vi "System und Gaseinstellung V2.vi"() -> ()   [LabVIEW 2020, in "System Einstellungen V2.lvlib"]
uses:
  System Einstellungen V2.lvlib
  Visualisierungs Elemente/String - Eingabefeld.ctl
  Gasflasche.ctl
  Gasflaschenkomponente.ctl
  Traegergas.ctl
  Visualisierungs Elemente/Button.ctl
  Optionen Eingabe.ctl
  Visualisierungs Elemente/Checkbox(boolsch).ctl
  Analysatoren.ctl
  Optionen.ctl
  Sprachverwaltung/FGV Aktion Tabelle zerlegen.ctl
  Passwortverwaltung/FGV Passwort Aktion.ctl
  Aktion FGV Gasbottledefinition.ctl
  Aktion FGV SystemEinstellungenV2.ctl
  Analysator Definition/FGV Analysator Definition Aktionen.ctl
  Aktioen FGV System.ctl
  AnalysatorDefinition.ctl
  Allgemein/allgemeine Sub-VIs.lvlib
  Sprachverwaltung/Sprachverwaltung.lvlib
  <vilib>/nisyscfg/nisyscfg.lvlib
  Passwortverwaltung/Passwort.lvlib
  Analysator Definition/Analysator Definition.lvlib
panel:
  in  "Registerkartenelement":T1(tab)
  in  "Werkseinstellung erstellen":T2 caption="Werkseinstellung"
  in  "Optionen Speichern":T2 caption="Speichern"
  in  "Neustart":T2
  in  "atm":dbl
  in  "mbar":dbl
  out "Zeit Steuerunge":timestamp caption="Aktuelle Zeit Steuerung:"
  out "Zeit Anlage":timestamp caption="Aktuelle Zeit Anlage:"
  in  "Systemzeit ändern":T2
  in  "Wartungsintervall:":sgl caption="Wartungsintervall" format="%#_5g"
  in  "Optionen":T3
  in  "Seriennummer":string caption="Seriennummer (fürs Protokoll)"
  in  "Type number (for Protocol)":string caption="Typennummer (fürs Protokoll)"
  in  "Analysator":T5="FT-IR"
  in  "Gasteiler Export":bool caption="Schaltfläche"
  in  "Gasteiler Importieren":bool caption="Schaltfläche"
  in  "Neuer Analysator":bool caption="Schaltfläche"
  in  "Name für Protokoll":string caption="Name (fürs Protokoll)"
  in  "Analysator löschen":bool caption="Schaltfläche"
  in  "Analysatoren Liste":i32(listbox) caption="Analyzer Definition"
  in  "Gasteiler Tabelle":i32(listbox) caption="Gas Divider Definition"
  in  "Neuer Gasteiler":bool caption="Schaltfläche"
  in  "Gasteiler Seriennummer":string caption="Seriennummer (fürs Protokoll)"
  in  "Gasteiler löschen":bool caption="Schaltfläche"
  in  "Gasteiler Type":string caption="Typennummer (fürs Protokoll)"
  in  "Gasteiler Name":string caption="Name"
  in  "Gasteiler Letzte Wartung":timestamp caption="Letzte Wartung" format="%<%d.%m.%Y>T"
  in  "Gasflaschenliste löschen":bool caption="Schaltfläche"
  in  "Gasflasche löschen":bool caption="Schaltfläche"
  in  "Gasflasche einfügen":bool caption="Schaltfläche"
  in  "Gasflasche ändern":bool caption="Schaltfläche"
  in  "Trägergas":T6="N2"
  in  "Komponente 5":T7={"Gasauswahl"="", "Konzentration IST"=0.0, "Einheit"="ppm", "Genauigkeit"=0.0} {"Konzentration IST" format="%#.4f"; "Genauigkeit" format="%#.1f"}
  in  "Komponente 4":T7={"Gasauswahl"="", "Konzentration IST"=0.0, "Einheit"="ppm", "Genauigkeit"=0.0} {"Konzentration IST" format="%#.4f"; "Genauigkeit" format="%#.1f"}
  in  "Komponente 3":T7={"Gasauswahl"="", "Konzentration IST"=0.0, "Einheit"="ppm", "Genauigkeit"=0.0} {"Konzentration IST" format="%#.4f"; "Genauigkeit" format="%#.1f"}
  in  "Komponente 2":T7={"Gasauswahl"="", "Konzentration IST"=0.0, "Einheit"="ppm", "Genauigkeit"=0.0} {"Konzentration IST" format="%#.4f"; "Genauigkeit" format="%#.1f"}
  in  "Komponente 1":T7={"Gasauswahl"="", "Konzentration IST"=0.0, "Einheit"="ppm", "Genauigkeit"=0.0} {"Konzentration IST" format="%#.4f"; "Genauigkeit" format="%#.1f"}
  in  "Gasflasche":T8={"Gasname für die Auswahl"="CH4", "Chargennummer"="D15442589", "Ablaufdatum"=timestamp(0 s since 1904-01-01)} {"Ablaufdatum" format="%<%d.%m.%Y>T"}
  in  "GF import":bool caption="Schaltfläche 2"
  in  "GF export":bool caption="Schaltfläche"
  in  "Gasflaschen Liste":i32(listbox)
  in  "Update Gas Selects":bool caption="Schaltfläche"
  in  "Gas Eingabe":T9 caption="Gasbezeichnung:"
  in  "Gas einfügen":bool caption="Schaltfläche"
  in  "Gas löschen":bool caption="Schaltfläche"
  in  "Gasauswahl":i32(listbox) caption="Gasauswahl:"
  # "Systemeinstellungen"
  # "Optionen"
  # "System Werkzeuge"
  # "Zeiteinstellung"
  # "Umrechner"
  # "Analysatorkonfiguration"
  # "Gasteilerkonfiguration"
  # "Gasflaschenkonfiguration"
  # "Gas"
  # "Konzentration"
  # "Einheit"
  # "Genauigkeit [%]"
  # "Gasflaschenliste"
  # "Gasdefinition"
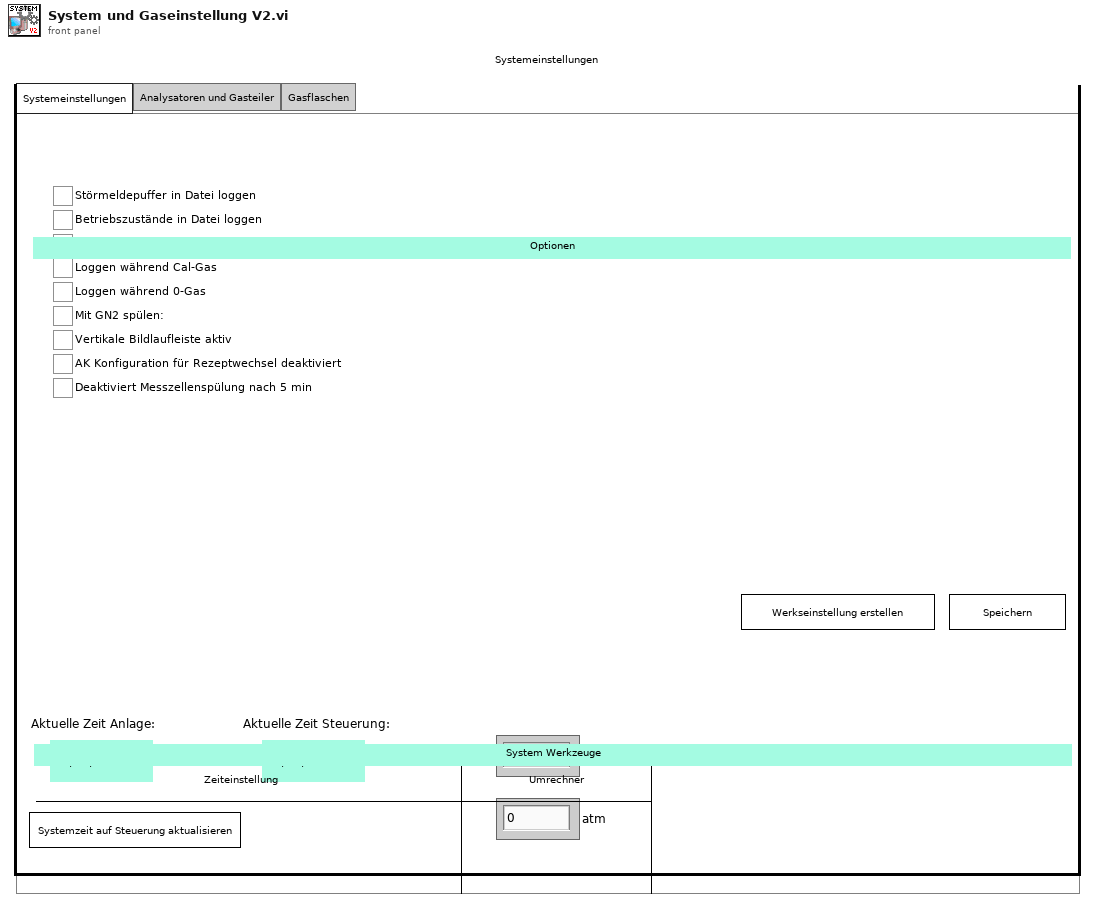
[diagram p1: front panel]
types:
  T1 = enum32{"Systemeinstellungen", "Analysatoren", "Gasflaschenkonfiguration", "Gasdefinition"}
  T2 = typedef "Button.ctl" = bool
  T3 = typedef "System Einstellungen V2.lvlib/Optionen Eingabe.ctl" = cluster{"Option 1":T4, "Option 2":T4, "Option 3":T4, "Option 4":T4, "Option 5":T4, "Option 6":T4, "Option 7":T4, "Option 8":T4, "Option 9":T4, "Option 10":T4, "Option 11":T4, "Option 12":T4, "Option 13":T4, "Option 14":T4, "Option 15":T4, "Option 16":T4, "Option 17":T4, "Option 18":T4, "Option 19":T4, "Option 20":T4, "Option 21":T4, "Option 22":T4, "Option 23":T4, "Option 24":T4, "Option 25":T4, "Option 26":T4, "Option 27":T4, "Option 28":T4, "Option 29":T4, "Option 30":T4, "Option 31":T4, "Option 32":T4, "Option 33":T4, "Option 34":T4, "Option 35":T4, "Option 36":T4, "Option 37":T4, "Option 38":T4, "Option 39":T4, "Option 40":T4, "Option 41":T4, "Option 42":T4, "Option 43":T4, "Option 44":T4, "Option 45":T4, "Option 46":T4, "Option 47":T4, "Option 48":T4, "Option 49":T4, "Option 50":T4, "Option 51":T4, "Option 52":T4, "Option 53":T4, "Option 54":T4, "Option 55":T4, "Option 56":T4, "Option 57":T4, "Option 58":T4, "Option 59":T4, "Option 60":T4}
  T4 = typedef "Checkbox(boolsch).ctl" = bool
  T5 = typedef "System Einstellungen V2.lvlib/Analysatoren.ctl" = string
  T6 = typedef "System Einstellungen V2.lvlib/Traegergas.ctl" = string
  T7 = typedef "System Einstellungen V2.lvlib/Gasflaschenkomponente.ctl" = cluster{"Gasauswahl":string, "Konzentration IST":dbl, "Einheit":string, "Genauigkeit":dbl}
  T8 = typedef "System Einstellungen V2.lvlib/Gasflasche.ctl" = cluster{"Gasname für die Auswahl":string, "Chargennummer":string, "Ablaufdatum":timestamp}
  T9 = typedef "String - Eingabefeld.ctl" = string
  T10 = typedef "Sprachverwaltung.lvlib/FGV Aktion Tabelle zerlegen.ctl" = enum16{"laden", "vereinzeln", "speichern"}
  T11 = enum8{"Enabled", "Disabled", "Disabled and Grayed Out"}
  T12 = typedef "Passwort.lvlib/FGV Passwort Aktion.ctl" = enum16{"prüfen", "setzen", "Initialisieren", "PW speichern", "lesen", "PW Änderung"}
  T13 = typedef "System Einstellungen V2.lvlib/Aktion FGV Gasbottledefinition.ctl" = enum16{"lesen", "schreiben", "löschen", "laden", "speichern", "exportieren", "importieren"}
  T14 = enum16{"lesen", "schreiben", "löschen", "laden", "speichern"}
  T15 = typedef "Analysator Definition.lvlib/FGV Analysator Definition Aktionen.ctl" = enum16{"lesen", "MB setzen", "MB KAL setzen", "laden"}
  T16 = typedef "System Einstellungen V2.lvlib/Aktion FGV SystemEinstellungenV2.ctl" = enum16{"lesen", "Analysatoren schreiben", "Analysator ändern", "Analysatoren löschen", "laden", "speichern", "Untertitel", "Analysatoren", "Neue Analysatoren", "Gasteiler schreiben", "Gasteiler ändern", "Gasteiler löschen", "Gasteiler", "Gasteiler exportieren", "Gasteiler importieren"}
  T17 = typedef "System Einstellungen V2.lvlib/Aktioen FGV System.ctl" = enum16{"lesen", "laden", "speichern", "Optionen schreiben", "Zeitstempel", "Reset BMP", "Reset SQP", "Wartung", "Werkseinstellung"}
  T18 = typedef "System Einstellungen V2.lvlib/Optionen.ctl" = cluster{"Störmeldep.":bool, "Betriebszustände":bool, "AK in ppm":bool, "log Cal-Gas":bool, "log 0-Gas":bool, "Durchflusssensor 0-5V":bool, "PNS?":bool, "Mit N2 spülen":bool, "TRE08":bool, "Amium 10-Fach":bool, "Verticale Scrollbar aktiv":bool, "Loggingtakt":bool, "AK Rezeptwechsel gleich wie MKS":bool, "NG ECO":bool}
  T19 = typedef "System Einstellungen V2.lvlib/Gasteiler.ctl" = cluster{"Gasteiler Name":string, "Gasteiler Type":string, "Gasteiler Seriennummer":string, "Gasteiler Letzte Wartung":timestamp}
  T20 = cluster{"GasteilerDefinitionsListe":T19[], "GasteilerDefinitionTextliste":string[][], "Gasteiler Strings And Values":cluster{"String":string, "Wert":string}[]}
  T21 = typedef "System Einstellungen V2.lvlib/AnalysatorDefinition.ctl" = cluster{"Analysator":string, "Name für Protokoll":string, "Type":string, "Seriennummer":string}
  T22 = typedef "LVComboBoxStrsAndValuesArrayTypeDef.ctl" = cluster{"String":string, "Value":string}[]
  T23 = cluster{"AnalysatorDefinitionListe":T21[], "AnalysatorDefinitionTextListe":string[][], "Analysatoren Strings And Values[]":T22}
  T24 = cluster{"Gasteiler Name":string, "Gasteiler Type":string, "Gasteiler Seriennummer":string, "Gasteiler Letzte Wartung":timestamp}
  T25 = typedef "System Einstellungen V2.lvlib/Gasflasche gesamt.ctl" = cluster{"Gasflasche":T8, "Trägergas":T6, "Komponenten":T7[]}
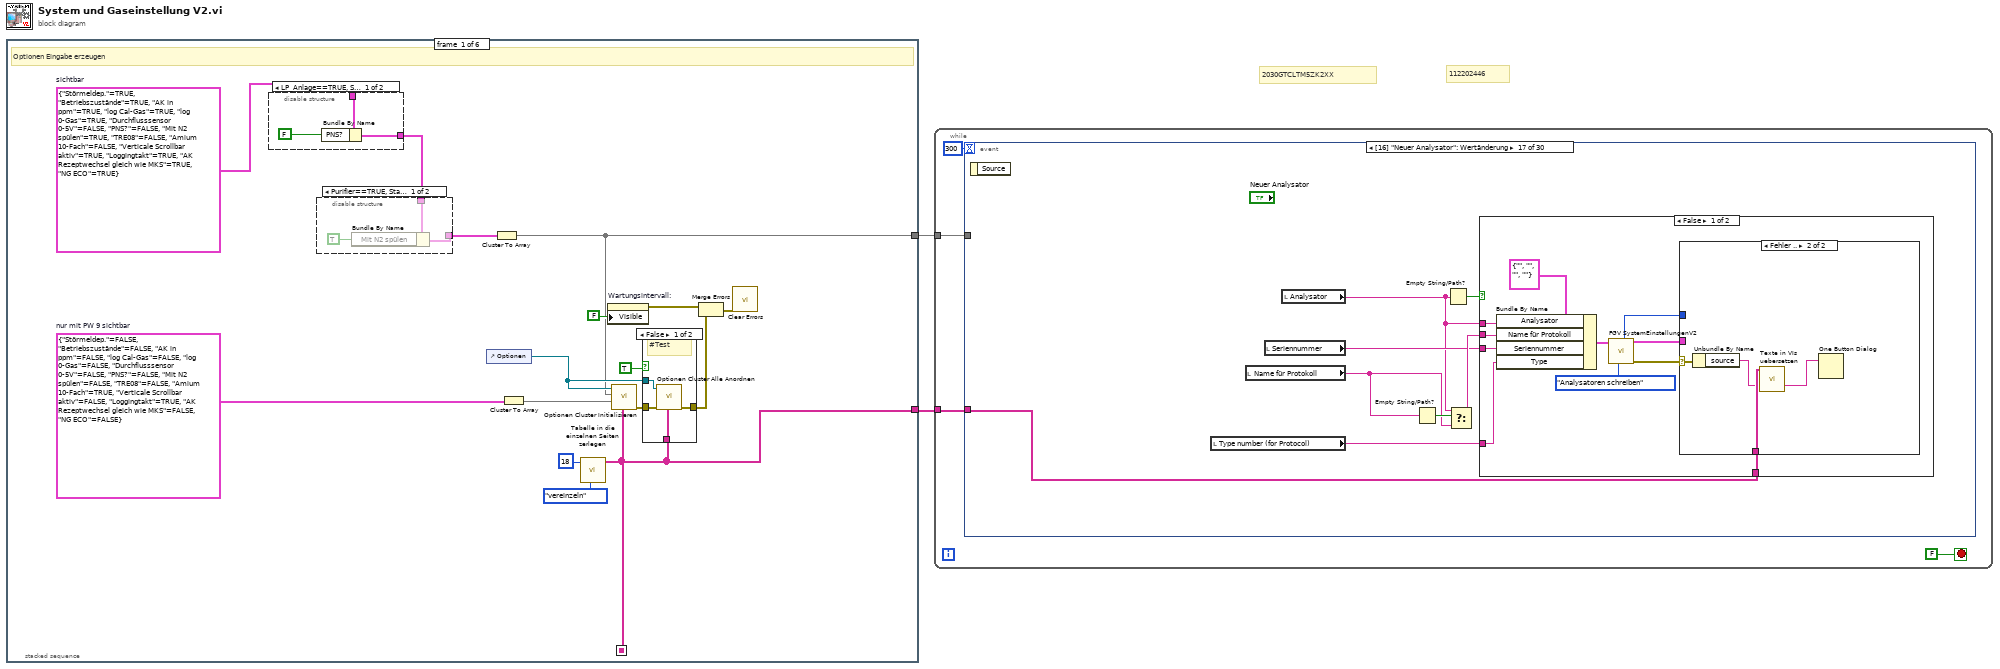
[diagram p0: block diagram]
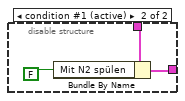
[diagram p2: hidden frame]
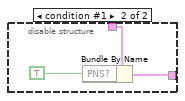
[diagram p3: hidden frame]
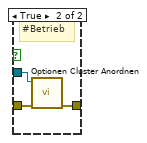
[diagram p4: hidden frame]
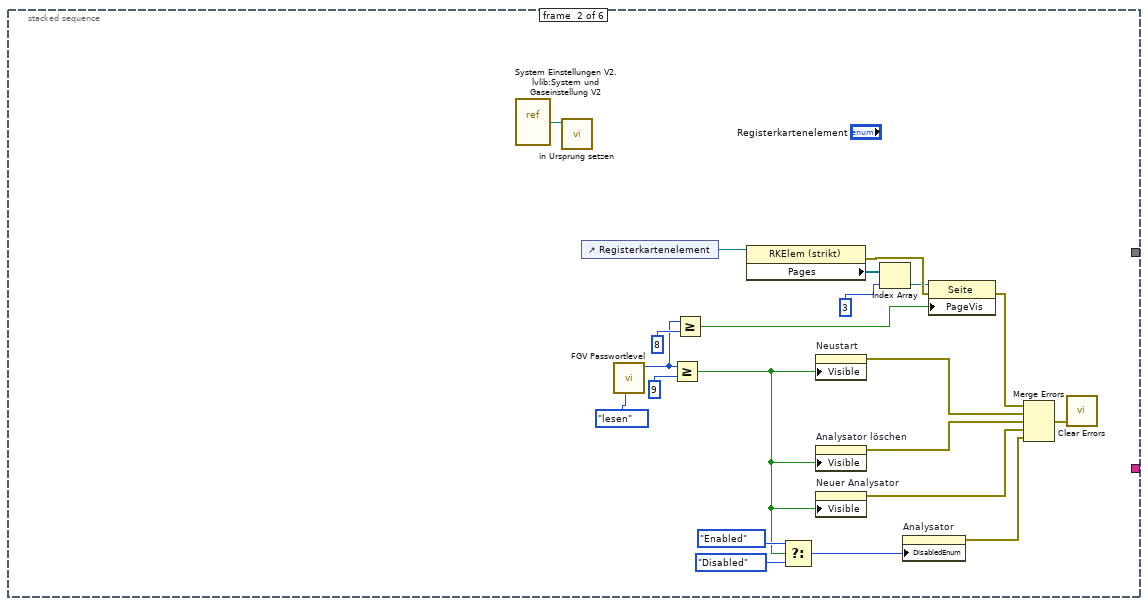
[diagram p5: hidden frame]
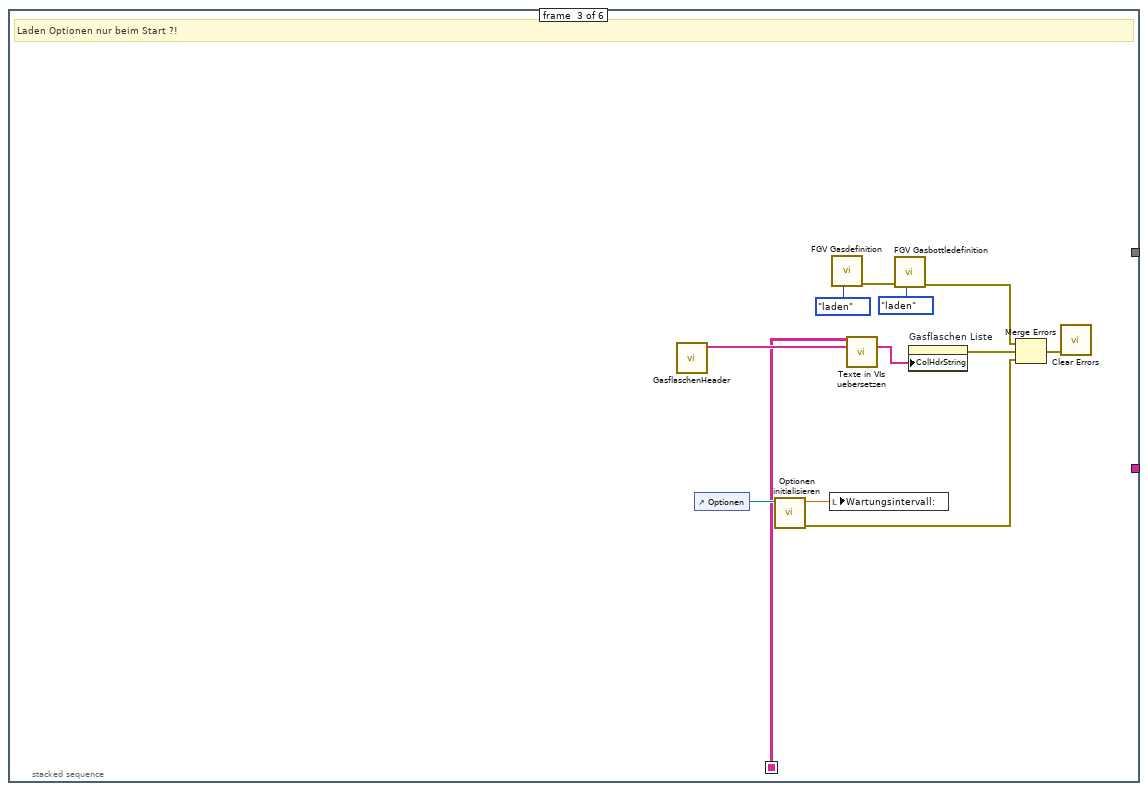
[diagram p6: hidden frame]
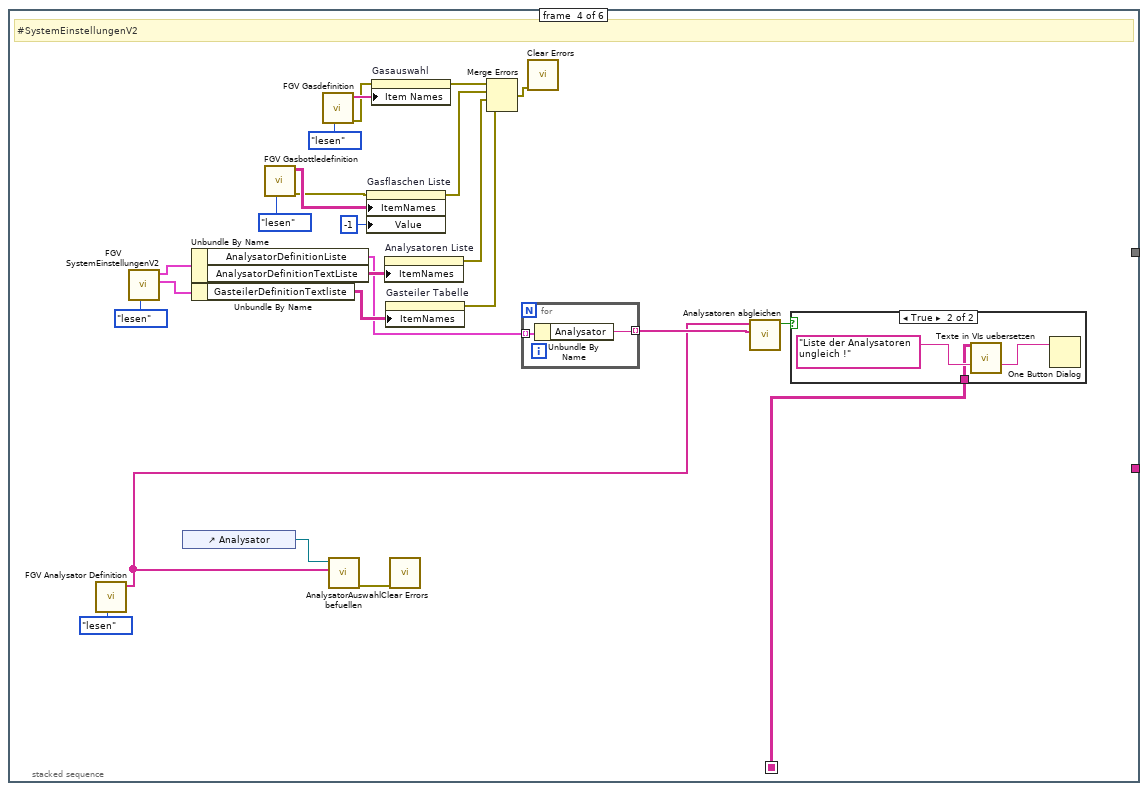
[diagram p7: hidden frame]
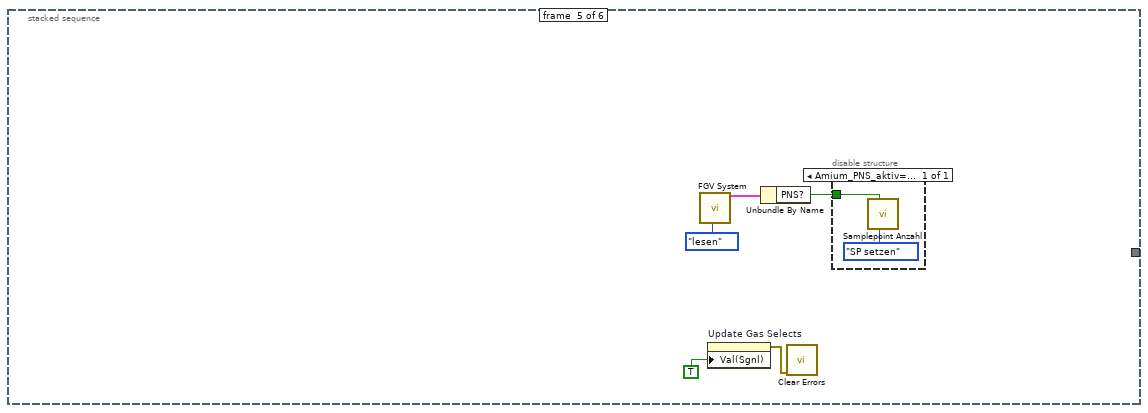
[diagram p9: hidden frame]
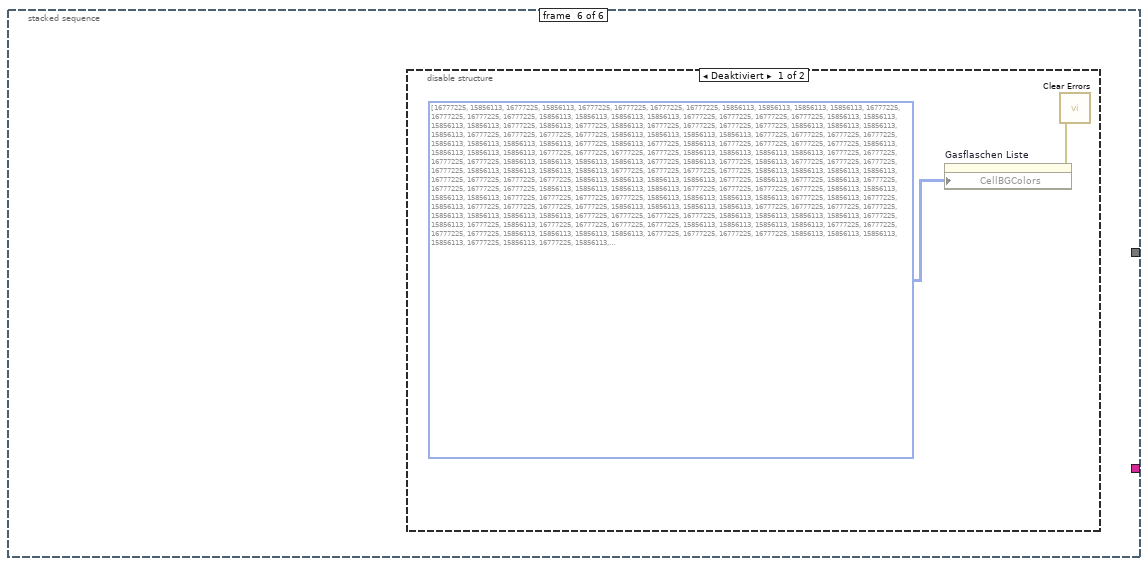
[diagram p10: hidden frame]
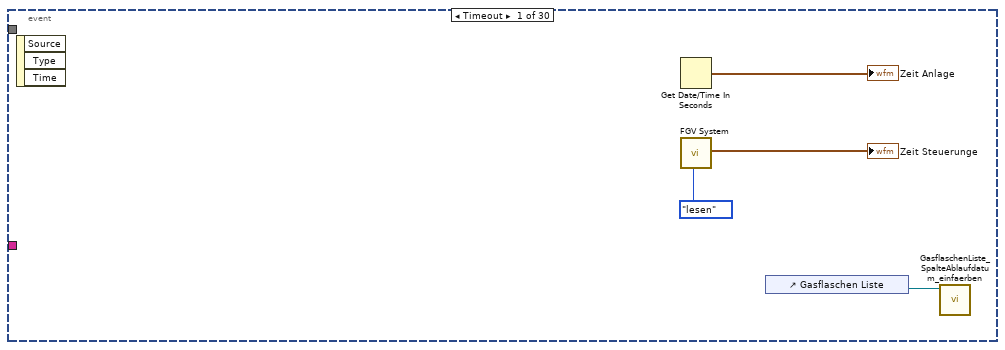
[diagram p12: hidden frame]
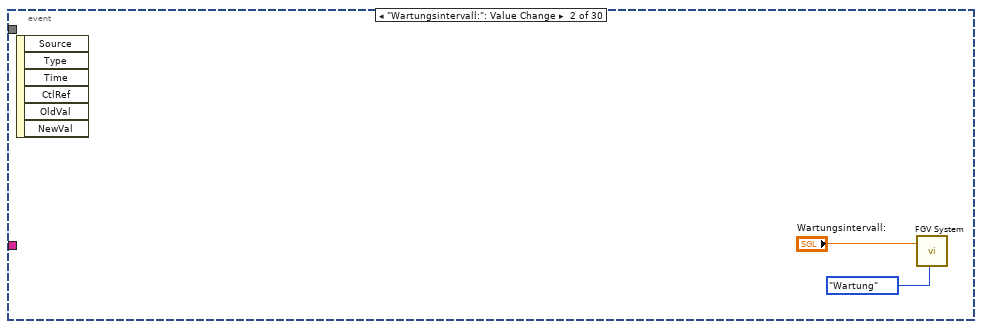
[diagram p13: hidden frame]
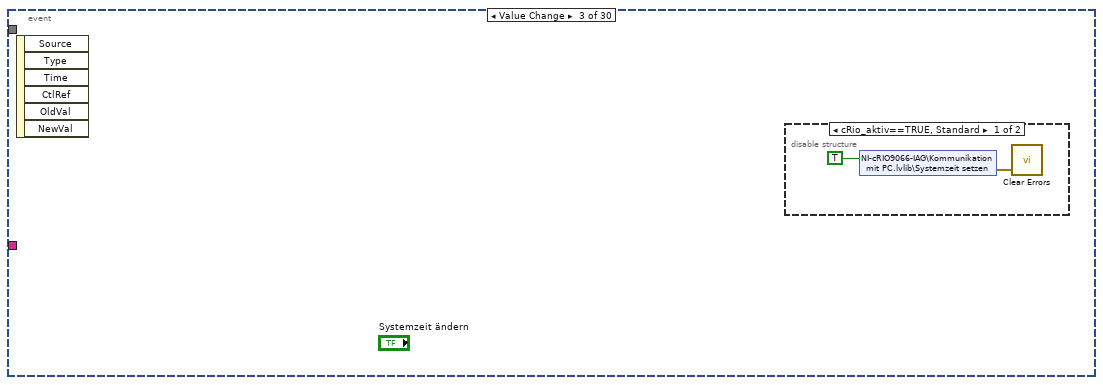
[diagram p14: hidden frame]
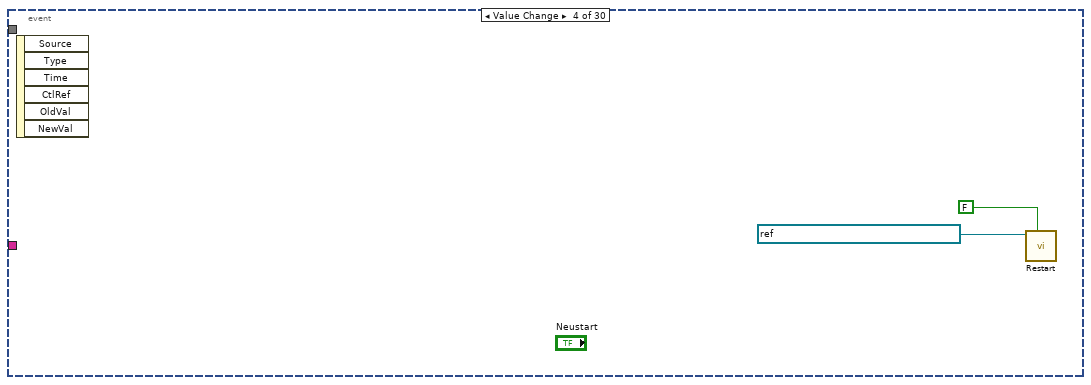
[diagram p16: hidden frame]
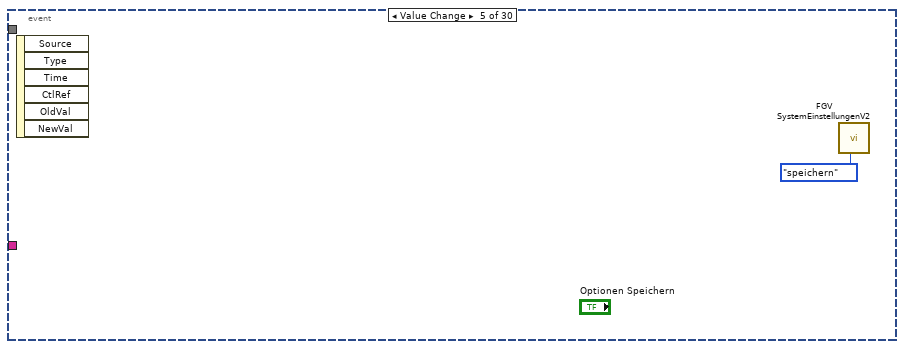
[diagram p17: hidden frame]
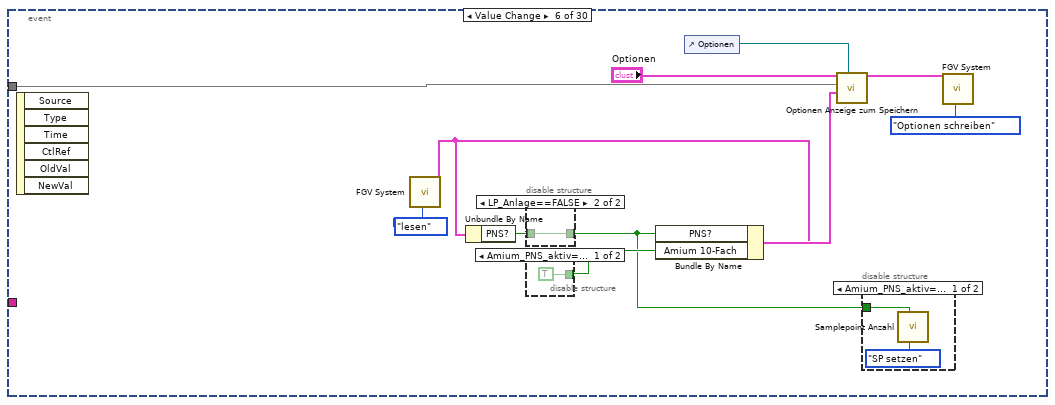
[diagram p18: hidden frame]
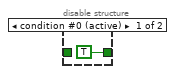
[diagram p19: hidden frame]
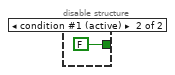
[diagram p20: hidden frame]
diagram:
  # "112202446"
  # "2030GTCLTM5ZK2XX"
  n1 = stacked-sequence {
    seq-local: [w3 _ _ _ _ _] -> [_ _ w59 w71 _ _]
    tunnel: [w14 _ _ _ _ _] -> w2
    tunnel: [w3 _ _ _ _ _] -> w1
    frame #0 {
      w12 = T18 {"Störmeldep."=FALSE, "Betriebszustände"=FALSE, "AK in ppm"=FALSE, "log Cal-Gas"=FALSE, "log 0-Gas"=FALSE, "Durchflusssensor 0-5V"=FALSE, "PNS?"=FALSE, "Mit N2 spülen"=FALSE, "TRE08"=FALSE, "Amium 10-Fach"=TRUE, "Verticale Scrollbar aktiv"=FALSE, "Loggingtakt"=TRUE, "AK Rezeptwechsel gleich wie MKS"=FALSE, "NG ECO"=FALSE}  # nur mit PW 9 sichtbar
      w11 = T18 {"Störmeldep."=TRUE, "Betriebszustände"=TRUE, "AK in ppm"=TRUE, "log Cal-Gas"=TRUE, "log 0-Gas"=TRUE, "Durchflusssensor 0-5V"=FALSE, "PNS?"=FALSE, "Mit N2 spülen"=TRUE, "TRE08"=FALSE, "Amium 10-Fach"=FALSE, "Verticale Scrollbar aktiv"=TRUE, "Loggingtakt"=TRUE, "AK Rezeptwechsel gleich wie MKS"=TRUE, "NG ECO"=TRUE}  # sichtbar
      # "Optionen Eingabe erzeugen"
      n2 = disable-structure shown="LP_Anlage==TRUE, Standard" {
        disable-tunnel: w11 -> [w27 w28]
        disable-tunnel: [w25 w29] -> w10
        frame condition #0 (active) {
          n3 = Bundle By Name(cluster=w27, "PNS?"=FALSE ("Störmeldepuffer")) -> (w25:T18)
        }
        frame condition #1 {
          n4 = Bundle By Name(cluster=w28, "PNS?"=TRUE ("Störmeldepuffer")) -> (w29:T18)
        }
      }
      n5 = disable-structure shown="Purifier==TRUE, Standard" {
        disable-tunnel: w10 -> [w21 w23]
        disable-tunnel: [w19 w22] -> w9
        frame condition #0 {
          n6 = Bundle By Name(cluster=w21, "Mit N2 spülen"=TRUE ("Störmeldepuffer")) -> (w19:T18)
        }
        frame condition #1 (active) {
          n7 = Bundle By Name(cluster=w23, "Mit N2 spülen"=FALSE ("Störmeldepuffer")) -> (w22:T18)
        }
      }
      n8 = control-ref of="Optionen"() -> (w17:refnum<vi>)
      n9 = Cluster To Array(cluster=w9) -> (array=w14:bool[])
      n10 = Cluster To Array(cluster=w12) -> (array=w13:bool[])
      n11 = call "Tabelle in die einzelnen Seiten zerlegen.vi"("Aktion"=FGV_Aktion_Tabelle_zerlegen."vereinzeln", "Index (Seite)"=18) -> ("Sprachliste"=w3:string[][])  [unwired: 7 in, 2 out]
      n12 = property on="Wartungsintervall:" class="DigWert (strikt)"("Visible"=FALSE ("Sichtbar")) -> (error out=w8:errorcluster)  [unwired: 2 in, 1 out]
      n13 = call "Optionen Cluster Initialisieren.vi"("Sprachliste"=w3, "PWL9"=w13, "sichtbar"=w14, "Cluster (Eingang)"=w17) -> ("error out"=w16:errorcluster)  [unwired: 5 in, 2 out]
      n14 = case shown="False" TRUE {
        tunnel: w17 -> [w32 w37]
        tunnel: w16 -> [w34 w36]
        tunnel: [w33 w35] -> w7
        tunnel: w3 -> [w31 _]
        frame False {
          # "#Test"
          n15 = call "Optionen Cluster Alle Anordnen.vi"("Sprachliste"=w31, "error in (no error)"=w34, "Cluster (Eingang)"=w32) -> ("error out"=w33:errorcluster)  [unwired: 7 in, 1 out]
        }
        frame True {
          # "#Betrieb"
          n16 = call "Optionen Cluster Anordnen.vi"("error in (no error)"=w36, "Cluster (Eingang)"=w37) -> ("error out"=w35:errorcluster)  [unwired: 8 in, 1 out]
        }
      }
      n17 = Merge Errors(w8, w7) -> (w6:errorcluster)
      n18 = call <vilib>:"Clear Errors.vi"("error in (no error)"=w6) -> ()  [unwired: 5 in, 2 out]
    }
    frame #1 {
      n19 = vi-ref "System Einstellungen V2.lvlib:System und Gaseinstellung V2.vi"() -> (w58:refnum<vi>)
      n20 = call "in Ursprung setzen.vi"("VI Referenz"=w58) -> ()  [unwired: 10 in, 1 out]
      n21 = control-ref of="Registerkartenelement"() -> (w52:refnum<vi>)
      n22 = call "FGV Passwortlevel.vi"("FGV Passwort Aktion"=FGV_Passwort_Aktion."lesen") -> ("aktueller Level"=w41:i16)  [unwired: 8 in, 2 out]
      n23 = Greater Or Equal?(x=w41, y=i16 9) -> (x >= y?=w43:bool)
      n24 = Greater Or Equal?(x=w41, y=i16 8) -> (x >= y?=w40:bool)
      n25 = property class="RKElem (strikt)"(reference=w52) -> (error out=w55:errorcluster, "Pages"=w54:refnum<vi>[])  [unwired: 1 in, 1 out]
      n26 = Select(t=T11."Enabled" ("Deaktiviert"), s=w43, f=T11."Disabled") -> (s? t:f=w39:T11)
      n27 = property on="Neustart" class="Bool."("Visible"=w43) -> (error out=w50:errorcluster)  [unwired: 2 in, 1 out]
      n28 = property on="Analysator löschen" class="Bool."("Visible"=w43) -> (error out=w47:errorcluster)  [unwired: 2 in, 1 out]
      n29 = property on="Neuer Analysator" class="Bool."("Visible"=w43) -> (error out=w46:errorcluster)  [unwired: 2 in, 1 out]
      n30 = Index Array(array=w54, index=3 ("Index")) -> (element=w53:refnum<vi>)
      n31 = property on="Analysator" class="KombiFeld (strikt)"("DisabledEnum"=w39) -> (error out=w38:errorcluster)  [unwired: 2 in, 1 out]
      n32 = property class="Seite"(reference=w53, error in=w55, "PageVis"=w40) -> (error out=w49:errorcluster)  [unwired: 1 out]
      n33 = Merge Errors(w49, w50, w47, w46, w38) -> (w48:errorcluster)
      n34 = call <vilib>:"Clear Errors.vi"("error in (no error)"=w48) -> ()  [unwired: 5 in, 2 out]
    }
    frame #2 {
      # "Laden Optionen nur beim Start ?!"
      n35 = call "GasflaschenHeader.vi"() -> ("Header"=w67:string[])  [unwired: 10 in, 1 out]
      n36 = control-ref of="Optionen"() -> (w65:refnum<vi>)
      n37 = call "Optionen initialisieren.vi"("Cluster (Eingang)"=w65) -> ("Fehler (Ausgang)"=w62:errorcluster, "Wartungsintervall:"=w64:sgl)  [unwired: 9 in]
      n38 = local write "Wartungsintervall:"(w64) -> ()
      n39 = call "FGV Gasdefinition.vi"("Aktion"=T14."laden") -> ("error out"=w68:errorcluster)  [unwired: 9 in, 1 out]
      n40 = call "Texte in VIs uebersetzen.vi"("Sprachliste"=w59, "String-Array zum Übersetzen"=w67) -> ("String-Array zum Übersetzen"=w66:string[])  [unwired: 9 in, 4 out]
      n41 = call "FGV Gasbottledefinition.vi"("Aktion"=Aktion_FGV_Gasbottledefinition."laden", "error in (no error)"=w68) -> ("error out"=w61:errorcluster)  [unwired: 7 in, 2 out]
      n42 = property on="Gasflaschen Liste" class="MehrSpaltFeld (strikt)"("ColHdrString"=w66) -> (error out=w63:errorcluster)  [unwired: 2 in, 1 out]
      n43 = Merge Errors(w61, w63, w62) -> (w60:errorcluster)
      n44 = call <vilib>:"Clear Errors.vi"("error in (no error)"=w60) -> ()  [unwired: 5 in, 2 out]
    }
    frame #3 {
      # "#SystemEinstellungenV2"
      n45 = call "FGV Analysator Definition.vi"("Aktionen"=FGV_Analysator_Definition_Aktionen."lesen") -> ("Analysatoren"=w72:string[])  [unwired: 6 in, 4 out]
      n46 = call "FGV SystemEinstellungenV2.vi"("Aktion"=Aktion_FGV_SystemEinstellungenV2."lesen") -> ("Gasteiler"=w85:T20, "Analysatoren"=w86:T23)  [unwired: 5 in, 4 out]
      n47 = control-ref of="Analysator"() -> (w75:refnum<vi>)
      n48 = Unbundle By Name(w86) -> ("AnalysatorDefinitionListe"=w83:T21[], "AnalysatorDefinitionTextListe"=w87:string[][])
      n49 = Unbundle By Name(w85) -> ("GasteilerDefinitionTextliste"=w84:string[][])
      n50 = call "FGV Gasbottledefinition.vi"("Aktion"=Aktion_FGV_Gasbottledefinition."lesen") -> ("error out"=w91:errorcluster, "Gasflaschen Text Liste gesamt"=w92:T6[][])  [unwired: 8 in, 1 out]
      n51 = call "FGV Gasdefinition.vi"("Aktion"=T14."lesen") -> ("error out"=w90:errorcluster, "Gase"=w94:string[])  [unwired: 9 in]
      n52 = call "AnalysatorAuswahl befuellen.vi"("Analysatoren"=w72, "Analysator Definition (Eingang)"=w75) -> ("error out"=w76:errorcluster)  [unwired: 9 in]
      n53 = property on="Gasflaschen Liste" class="MehrSpaltFeld (strikt)"(error in=w91, "ItemNames"=w92, "Value"=-1 ("Gasflaschen Liste")) -> (error out=w79:errorcluster)  [unwired: 1 in, 1 out]
      n54 = property on="Gasauswahl" class="Listenfeld (strikt)"(error in=w90, "Item Names"=w94) -> (error out=w81:errorcluster)  [unwired: 1 in, 1 out]
      n55 = property on="Analysatoren Liste" class="MehrSpaltFeld (strikt)"("ItemNames"=w87) -> (error out=w78:errorcluster)  [unwired: 2 in, 1 out]
      n56 = property on="Gasteiler Tabelle" class="MehrSpaltFeld (strikt)"("ItemNames"=w84) -> (error out=w77:errorcluster)  [unwired: 2 in, 1 out]
      n57 = call <vilib>:"Clear Errors.vi"("error in (no error)"=w76) -> ()  [unwired: 5 in, 2 out]
      n58 = Merge Errors(w81, w79, w78, w77) -> (w80:errorcluster)
      n59 = for {
        tunnel: w83 -> [w100] mode=indexing
        tunnel: [w99] -> w82 mode=indexing
        n60 = Unbundle By Name(w100) -> ("Analysator"=w99:string)
      }
      n61 = call <vilib>:"Clear Errors.vi"("error in (no error)"=w80) -> ()  [unwired: 5 in, 2 out]
      n62 = call "Analysatoren abgleichen.vi"("Analysatorliste"=w82, "Analysatoren"=w72) -> ("x != y?"=w73:bool)  [unwired: 9 in]
      n63 = case shown="True" w73 {
        tunnel: w71 -> [_ w96]
        frame False {
        }
        frame True {
          n64 = call "Texte in VIs uebersetzen.vi"("Sprachliste"=w96, "String zum Übersetzen"="Liste der Analysatoren ungleich !" ("Nachricht")) -> ("String zum Übersetzen"=w97:string)  [unwired: 9 in, 4 out]
          n65 = One Button Dialog(message=w97) -> ()  [unwired: 1 in, 1 out]
        }
      }
    }
    frame #4 {
      n66 = call "FGV System.vi"("Aktionen"=Aktioen_FGV_System."lesen") -> ("Optionen"=w103:T18)  [unwired: 12 in, 6 out]
      n67 = property on="Update Gas Selects" class="Bool. (strikt)"("Val(Sgnl)"=TRUE ("Wert (signalisierend)")) -> (error out=w105:errorcluster)  [unwired: 2 in, 1 out]
      n68 = Unbundle By Name(w103) -> ("PNS?"=w102:bool)
      n69 = call <vilib>:"Clear Errors.vi"("error in (no error)"=w105) -> ()  [unwired: 5 in, 2 out]
      n70 = disable-structure shown="Amium_PNS_aktiv==FALSE, Standard" {
        disable-tunnel: w102 -> [w106]
        frame condition #0 (active) {
          n71 = call "Samplepoint Anzahl.vi"("Aktion"=enum16{"lesen", "Ref schreiben", "SP setzen"}."SP setzen", "PNS aktiv"=w106) -> ()  [unwired: 8 in, 2 out]
        }
      }
    }
    frame #5 {
      n72 = disable-structure shown="Deaktiviert" {
        frame Disabled {
          n73 = property on="Gasflaschen Liste" class="MehrSpaltFeld (strikt)"("CellBGColors"=u32[][] [[16777225, 15856113, 16777225, 15856113, 16777225, 16777225, 16777225, 16777225, 15856113, 15856113, 15856113, 15856113, 16777225, 16777225, 16777225, 16777225, 15856113, 15856113, 15856113, 15856113, 16777225, 16777225, 16777225, 16777225, 15856113, 15856113, 15856113, 15856113], [16777225, 15856113, 16777225, 15856113, 16777225, 16777225, 16777225, 16777225, 15856113, 15856113, 15856113, 15856113, 16777225, 16777225, 16777225, 16777225, 15856113, 15856113, 15856113, 15856113, 16777225, 16777225, 16777225, 16777225, 15856113, 15856113, 15856113, 15856113], [16777225, 15856113, 16777225, 15856113, 16777225, 16777225, 16777225, 16777225, 15856113, 15856113, 15856113, 15856113, 16777225, 16777225, 16777225, 16777225, 15856113, 15856113, 15856113, 15856113, 16777225, 16777225, 16777225, 16777225, 15856113, 15856113, 15856113, 15856113], [16777225, 15856113, 16777225, 15856113, 16777225, 16777225, 16777225, 16777225, 15856113, 15856113, 15856113, 15856113, 16777225, 16777225, 16777225, 16777225, 15856113, 15856113, 15856113, 15856113, 16777225, 16777225, 16777225, 16777225, 15856113, 15856113, 15856113, 15856113], [16777225, 15856113, 16777225, 15856113, 16777225, 16777225, 16777225, 16777225, 15856113, 15856113, 15856113, 15856113, 16777225, 16777225, 16777225, 16777225, 15856113, 15856113, 15856113, 15856113, 16777225, 16777225, 16777225, 16777225, 15856113, 15856113, 15856113, 15856113], [16777225, 15856113, 16777225, 15856113, 16777225, 16777225, 16777225, 16777225, 15856113, 15856113, 15856113, 15856113, 16777225, 16777225, 16777225, 16777225, 15856113, 15856113, 15856113, 15856113, 16777225, 16777225, 16777225, 16777225, 15856113, 15856113, 15856113, 15856113], [16777225, 15856113, 16777225, 15856113, 16777225, 16777225, 16777225, 16777225, 15856113, 15856113, 15856113, 15856113, 16777225, 16777225, 16777225, 16777225, 15856113, 15856113, 15856113, 15856113, 16777225, 16777225, 16777225, 16777225, 15856113, 15856113, 15856113, 15856113], [16777225, 15856113, 16777225, 15856113, 16777225, 16777225, 16777225, 16777225, 15856113, 15856113, 15856113, 15856113, 16777225, 16777225, 16777225, 16777225, 15856113, 15856113, 15856113, 15856113, 16777225, 16777225, 16777225, 16777225, 15856113, 15856113, 15856113, 15856113], [16777225, 15856113, 16777225, 15856113, 16777225, 16777225, 16777225, 16777225, 15856113, 15856113, 15856113, 15856113, 16777225, 16777225, 16777225, 16777225, 15856113, 15856113, 15856113, 15856113, 16777225, 16777225, 16777225, 16777225, 15856113, 15856113, 15856113, 15856113], [16777225, 15856113, 16777225, 15856113, 16777225, 16777225, 16777225, 16777225, 15856113, 15856113, 15856113, 15856113, 16777225, 16777225, 16777225, 16777225, 15856113, 15856113, 15856113, 15856113, 16777225, 16777225, 16777225, 16777225, 15856113, 15856113, 15856113, 15856113], [16777225, 15856113, 16777225, 15856113, 16777225, 16777225, 16777225, 16777225, 15856113, 15856113, 15856113, 15856113, 16777225, 16777225, 16777225, 16777225, 15856113, 15856113, 15856113, 15856113, 16777225, 16777225, 16777225, 16777225, 15856113, 15856113, 15856113, 15856113], [16777225, 15856113, 16777225, 15856113, 16777225, 16777225, 16777225, 16777225, 15856113, 15856113, 15856113, 15856113, 16777225, 16777225, 16777225, 16777225, 15856113, 15856113, 15856113, 15856113, 16777225, 16777225, 16777225, 16777225, 15856113, 15856113, 15856113, 15856113], [16777225, 15856113, 16777225, 15856113, 16777225, 16777225, 16777225, 16777225, 15856113, 15856113, 15856113, 15856113, 16777225, 16777225, 16777225, 16777225, 15856113, 15856113, 15856113, 15856113, 16777225, 16777225, 16777225, 16777225, 15856113, 15856113, 15856113, 15856113], [16777225, 15856113, 16777225, 15856113, 16777225, 16777225, 16777225, 16777225, 15856113, 15856113, 15856113, 15856113, 16777225, 16777225, 16777225, 16777225, 15856113, 15856113, 15856113, 15856113, 16777225, 16777225, 16777225, 16777225, 15856113, 15856113, 15856113, 15856113], [16777225, 15856113, 16777225, 15856113, 16777225, 16777225, 16777225, 16777225, 15856113, 15856113, 15856113, 15856113, 16777225, 16777225, 16777225, 16777225, 15856113, 15856113, 15856113, 15856113, 16777225, 16777225, 16777225, 16777225, 15856113, 15856113, 15856113, 15856113], [16777225, 15856113, 16777225, 15856113, 16777225, 16777225, 16777225, 16777225, 15856113, 15856113, 15856113, 15856113, 16777225, 16777225, 16777225, 16777225, 15856113, 15856113, 15856113, 15856113, 16777225, 16777225, 16777225, 16777225, 15856113, 15856113, 15856113, 15856113], [16777225, 15856113, 16777225, 15856113, 16777225, 16777225, 16777225, 16777225, 15856113, 15856113, 15856113, 15856113, 16777225, 16777225, 16777225, 16777225, 15856113, 15856113, 15856113, 15856113, 16777225, 16777225, 16777225, 16777225, 15856113, 15856113, 15856113, 15856113], [16777225, 15856113, 16777225, 15856113, 16777225, 16777225, 16777225, 16777225, 15856113, 15856113, 15856113, 15856113, 16777225, 16777225, 16777225, 16777225, 15856113, 15856113, 15856113, 15856113, 16777225, 16777225, 16777225, 16777225, 15856113, 15856113, 15856113, 15856113], [16777225, 15856113, 16777225, 15856113, 16777225, 16777225, 16777225, 16777225, 15856113, 15856113, 15856113, 15856113, 16777225, 16777225, 16777225, 16777225, 15856113, 15856113, 15856113, 15856113, 16777225, 16777225, 16777225, 16777225, 15856113, 15856113, 15856113, 15856113], [16777225, 15856113, 16777225, 15856113, 16777225, 16777225, 16777225, 16777225, 15856113, 15856113, 15856113, 15856113, 16777225, 16777225, 16777225, 16777225, 15856113, 15856113, 15856113, 15856113, 16777225, 16777225, 16777225, 16777225, 15856113, 15856113, 15856113, 15856113], [16777225, 15856113, 16777225, 15856113, 16777225, 16777225, 16777225, 16777225, 15856113, 15856113, 15856113, 15856113, 16777225, 16777225, 16777225, 16777225, 15856113, 15856113, 15856113, 15856113, 16777225, 16777225, 16777225, 16777225, 15856113, 15856113, 15856113, 15856113], [16777225, 15856113, 16777225, 15856113, 16777225, 16777225, 16777225, 16777225, 15856113, 15856113, 15856113, 15856113, 16777225, 16777225, 16777225, 16777225, 15856113, 15856113, 15856113, 15856113, 16777225, 16777225, 16777225, 16777225, 15856113, 15856113, 15856113, 15856113]] ("Zellengruppen:Hintergrundfarben")) -> (error out=w108:errorcluster)  [unwired: 2 in, 1 out]
          n74 = call <vilib>:"Clear Errors.vi"("error in (no error)"=w108) -> ()  [unwired: 5 in, 2 out]
        }
        frame Enabled {
        }
      }
    }
  }
  n75 = while {
    tunnel: w2 -> [w111]
    tunnel: w1 -> [w110]
    stop <- FALSE stop-if-true
    n76 = event shown="[16] \"Neuer Analysator\": Wertänderung" {
      selector: _ -> [_ _ _ _ _ _ _ _ _ _ _ _ _ _ _ _ _ _ _ _ _ _ _ _ _ _ _ _ _ _]
      dyn-events: _ -> [_ _ _ _ _ _ _ _ _ _ _ _ _ _ _ _ _ _ _ _ _ _ _ _ _ _ _ _ _ _]
      timeout: 300 -> [_ _ _ _ _ _ _ _ _ _ _ _ _ _ _ _ _ _ _ _ _ _ _ _ _ _ _ _ _ _]
      tunnel: w111 -> [_ _ _ _ _ w132 _ _ _ _ _ _ _ _ _ _ _ _ _ _ _ _ _ _ _ _ _ _ _ _]
      tunnel: w110 -> [_ _ _ _ _ _ _ _ _ _ w169 w218 w246 _ w288 w316 w358 _ w397 w429 w456 _ _ w489 w502 w525 w547 w588 _ w615]
      event Timeout {
        n77 = event-data() -> ()  [unwired: 1 in, 3 out]
        n78 = Get Date/Time In Seconds() -> (seconds since 1Jan1904=→"Zeit Anlage":timestamp)
        n79 = call "FGV System.vi"("Aktionen"=Aktioen_FGV_System."lesen") -> ("Zeitstempel"=→"Zeit Steuerunge":timestamp)  [unwired: 12 in, 6 out]
        n80 = control-ref of="Gasflaschen Liste"() -> (w114:refnum<vi>)
        n81 = call "GasflaschenListe_SpalteAblaufdatum_einfaerben.vi"("MehrspaltigesListenfeld (Eingang)"=w114) -> ()  [unwired: 11 in]
      }
      event "Wartungsintervall:": Value Change {
        n82 = event-data() -> ()  [unwired: 1 in, 6 out]
        n83 = call "FGV System.vi"("Wartungsintervall:"="Wartungsintervall:", "Aktionen"=Aktioen_FGV_System."Wartung") -> ()  [unwired: 11 in, 7 out]
      }
      event Value Change {
        n84 = event-data() -> ()  [unwired: 1 in, 6 out]
        n85 = disable-structure shown="cRio_aktiv==TRUE, Standard" {
          frame condition #0 (active) {
            n86 = shared-variable "NI-cRIO9066-IAG\\Kommunikation mit PC.lvlib\\Systemzeit setzen"(TRUE ("Systemzeit setzen")) -> (error out=w120:errorcluster)  [unwired: 1 in]
            n87 = call <vilib>:"Clear Errors.vi"("error in (no error)"=w120) -> ()  [unwired: 5 in, 2 out]
          }
          frame condition #1 {
          }
        }
      }
      event Value Change {
        n88 = event-data() -> ()  [unwired: 1 in, 6 out]
        n89 = call <vilib>:"Restart.vi"("Wait Until Complete (T)"=FALSE, "Session in"=refnum<k21> "NI-cRIO-9066-IAG (192.168.14.14)") -> ()  [unwired: 7 in, 3 out]
      }
      event Value Change {
        n90 = event-data() -> ()  [unwired: 1 in, 6 out]
        n91 = call "FGV SystemEinstellungenV2.vi"("Aktion"=Aktion_FGV_SystemEinstellungenV2."speichern") -> ()  [unwired: 5 in, 6 out]
      }
      event Value Change {
        n92 = event-data() -> ()  [unwired: 1 in, 6 out]
        n93 = call "FGV System.vi"("Aktionen"=Aktioen_FGV_System."lesen") -> ("Optionen"=w126:T18)  [unwired: 12 in, 6 out]
        n94 = Unbundle By Name(w126) -> ("PNS?"=w125:bool)
        n95 = disable-structure shown="LP_Anlage==FALSE" {
          disable-tunnel: [TRUE ("Störmeldepuffer") w137] -> w127
          disable-tunnel: w125 -> [_ w137]
          frame condition #0 (active) {
          }
          frame condition #1 {
          }
        }
        n96 = disable-structure shown="Amium_PNS_aktiv==TRUE" {
          disable-tunnel: [TRUE ("Störmeldepuffer") FALSE ("Amium 10-Fach")] -> w128
          frame condition #0 {
          }
          frame condition #1 (active) {
          }
        }
        n97 = Bundle By Name(cluster=w126, "PNS?"=w127, "Amium 10-Fach"=w128) -> (w131:T18)
        n98 = control-ref of="Optionen"() -> (w130:refnum<vi>)
        n99 = call "Optionen Anzeige zum Speichern.vi"(7:"Optionen Anzeige (Eingang)"=w130, "Optionen fix"=w131, "sichtbar"=w132, 11:"Optionen Anzeige (Eingang)"="Optionen") -> ("Optionen out"=w134:T18)  [unwired: 6 in, 1 out]
        n100 = disable-structure shown="Amium_PNS_aktiv==FALSE" {
          disable-tunnel: w127 -> [w140 _]
          frame condition #0 (active) {
            n101 = call "Samplepoint Anzahl.vi"("Aktion"=enum16{"lesen", "Ref schreiben", "SP setzen"}."SP setzen", "PNS aktiv"=w140) -> ()  [unwired: 8 in, 2 out]
          }
          frame condition #1 {
          }
        }
        n102 = call "FGV System.vi"("Optionen"=w134, "Aktionen"=Aktioen_FGV_System."Optionen schreiben") -> ()  [unwired: 11 in, 7 out]
      }
      event "mbar": Value Change {
        n103 = event-data() -> ()  [unwired: 1 in, 6 out]
        n104 = Divide(x="mbar", y=1013.25) -> (x/y=w142:dbl)
        n105 = local write "atm"(w142) -> ()
      }
      event "atm": Value Change {
        n106 = event-data() -> ()  [unwired: 1 in, 6 out]
        n107 = Multiply(x="atm", y=1013.25) -> (x*y=w145:dbl)
        n108 = local write "mbar"(w145) -> ()
      }
      event Value Change {
        n109 = event-data() -> ()  [unwired: 1 in, 6 out]
        n110 = call "FGV System.vi"("Werkseinstellung erstellen"=T2 TRUE, "Aktionen"=Aktioen_FGV_System."Werkseinstellung") -> ("error out"=w155:errorcluster)  [unwired: 11 in, 6 out]
        n111 = control-ref of="Optionen"() -> (w149:refnum<vi>)
        n112 = call "Werkseinstellung erstellen.vi"("error in (no error)"=w155) -> ("error out"=w151:errorcluster)  [unwired: 10 in]
        n113 = call "Optionen initialisieren.vi"("error in (no error)"=w151, "Cluster (Eingang)"=w149) -> ("Fehler (Ausgang)"=w150:errorcluster, "Wartungsintervall:"=w148:sgl)  [unwired: 8 in]
        n114 = local write "Wartungsintervall:"(w148) -> ()
        n115 = property on="Werkseinstellung erstellen" class="Bool."(error in=w150, "Visible"=FALSE ("Sichtbar")) -> (error out=w152:errorcluster)  [unwired: 1 in, 1 out]
        n116 = call <vilib>:"Clear Errors.vi"("error in (no error)"=w152) -> ()  [unwired: 5 in, 2 out]
      }
      event "Gasteiler Tabelle": Value Change {
        n117 = event-data() -> ()  [unwired: 1 in, 1 out]
        n118 = call "FGV SystemEinstellungenV2.vi"("Aktion"=Aktion_FGV_SystemEinstellungenV2."lesen") -> ("Gasteiler"=w160:T20)  [unwired: 5 in, 5 out]
        n119 = Unbundle By Name(w160) -> ("GasteilerDefinitionsListe"=w161:T19[])
        n120 = Index Array(array=w161, index="Gasteiler Tabelle") -> (element=w163:T19)
        n121 = Unbundle By Name(w163) -> ("Gasteiler Name"=w162:string, "Gasteiler Type"=w159:string, "Gasteiler Seriennummer"=w158:string, "Gasteiler Letzte Wartung"=w157:timestamp)
        n122 = local write "Gasteiler Name"(w162) -> ()
        n123 = local write "Gasteiler Type"(w159) -> ()
        n124 = local write "Gasteiler Seriennummer"(w158) -> ()
        n125 = local write "Gasteiler Letzte Wartung"(w157) -> ()
      }
      event "Gasteiler Type", "Gasteiler Seriennummer", "Gasteiler Letzte Wartung": Value Change {
        n126 = event-data() -> ()  [unwired: 1 in, 1 out]
        n127 = call "FGV SystemEinstellungenV2.vi"("Aktion"=Aktion_FGV_SystemEinstellungenV2."lesen") -> ("Gasteiler"=w167:T20)  [unwired: 5 in, 5 out]
        n128 = local read "Gasteiler Name"() -> (w168:string)
        n129 = Unbundle By Name(w167) -> ("GasteilerDefinitionsListe"=w170:T19[])
        n130 = for {
          tunnel: w170 -> [w217] mode=indexing
          tunnel: w168 -> [w215]
          tunnel: [w214] -> w166
          stop <- w214 stop-if-true
          n131 = Unbundle By Name(w217) -> ("Gasteiler Name"=w216:string)
          n132 = Equal?(x=w215, y=w216) -> (x = y?=w214:bool)
        }
        n133 = case shown="True" w166 {
          tunnel: w169 -> [_ w172]
          tunnel: w168 -> [_ w173]
          frame False {
          }
          frame True {
            n134 = call "Texte in VIs uebersetzen.vi"("Sprachliste"=w172, "String zum Übersetzen"="Änderungen speichern?" ("Nachricht")) -> ("String zum Übersetzen"=w175:string)  [unwired: 9 in, 4 out]
            n135 = call "Texte in VIs uebersetzen.vi"("Sprachliste"=w172, "String zum Übersetzen"="Ja" ("Text für T-Schaltfläche (\"OK\")")) -> ("String zum Übersetzen"=w176:string)  [unwired: 9 in, 4 out]
            n136 = call "Texte in VIs uebersetzen.vi"("Sprachliste"=w172, "String zum Übersetzen"="Nein" ("Text für F-Schaltfläche (\"Abbrechen\")")) -> ("String zum Übersetzen"=w177:string)  [unwired: 9 in, 4 out]
            n137 = Two Button Dialog(message=w175, 1:w177, 2:w176) -> (T button?=w174:bool)
            n138 = case shown="True" w174 {
              tunnel: w173 -> [_ w182]
              tunnel: w172 -> [_ w181]
              frame False {
              }
              frame True {
                n139 = Empty String/Path?(string/path=w182) -> (empty?=w189:bool)
                n140 = Empty String/Path?(string/path="Gasteiler Type") -> (empty?=w190:bool)
                n141 = Select(t="Gasteiler Type", s=w189, f=w182) -> (s? t:f=w186:string)
                n142 = Select(t=w182, s=w190, f="Gasteiler Type") -> (s? t:f=w184:string)
                n143 = Empty String/Path?(string/path=w186) -> (empty?=w187:bool)
                n144 = case shown="False" w187 {
                  tunnel: w186 -> [w199 _]
                  tunnel: w184 -> [w198 _]
                  tunnel: "Gasteiler Seriennummer" -> [w197 _]
                  tunnel: "Gasteiler Letzte Wartung" -> [w196 _]
                  tunnel: w181 -> [w192 _]
                  frame False {
                    n145 = Bundle("Gasteiler Name"=w199, "Gasteiler Type"=w198, "Gasteiler Seriennummer"=w197, "Gasteiler Letzte Wartung"=w196) -> (w195:T24)  [unwired: 1 in]
                    n146 = call "FGV SystemEinstellungenV2.vi"("Aktion"=Aktion_FGV_SystemEinstellungenV2."Gasteiler ändern", "Gasteiler definition"=w195) -> ("error out"=w191:errorcluster, "Gasteiler"=w194:T20, "Index Neuer Gasteiler"=w193:i32)  [unwired: 4 in, 3 out]
                    n147 = case shown="Fehler .." w191 {
                      selector: w191 -> [_ w213]
                      tunnel: w194 -> [w202 _]
                      tunnel: w193 -> [w201 _]
                      tunnel: w192 -> [_ w210]
                      frame No Error {
                        n148 = stacked-sequence {
                          tunnel: w202 -> [w204 _]
                          tunnel: w201 -> [_ w209]
                          frame #0 {
                            n149 = Unbundle By Name(w204) -> ("GasteilerDefinitionTextliste"=w203:string[][])
                            n150 = call "FGV SystemEinstellungenV2.vi"("Aktion"=Aktion_FGV_SystemEinstellungenV2."speichern") -> ("error out"=w206:errorcluster)  [unwired: 5 in, 5 out]
                            n151 = property on="Gasteiler Tabelle" class="MehrSpaltFeld (strikt)"(error in=w206, "ItemNames"=w203) -> (error out=w205:errorcluster)  [unwired: 1 in, 1 out]
                            n152 = call <vilib>:"Clear Errors.vi"("error in (no error)"=w205) -> ()  [unwired: 5 in, 2 out]
                          }
                          frame #1 {
                            n153 = property on="Gasteiler Tabelle" class="MehrSpaltFeld (strikt)"("Val(Sgnl)"=w209) -> (error out=w208:errorcluster)  [unwired: 2 in, 1 out]
                            n154 = call <vilib>:"Clear Errors.vi"("error in (no error)"=w208) -> ()  [unwired: 5 in, 2 out]
                          }
                        }
                      }
                      frame Error {
                        n155 = Unbundle By Name(w213) -> ("source"=w212:string)
                        n156 = call "Texte in VIs uebersetzen.vi"("Sprachliste"=w210, "String zum Übersetzen"=w212) -> ("String zum Übersetzen"=w211:string)  [unwired: 9 in, 4 out]
                        n157 = One Button Dialog(message=w211) -> ()  [unwired: 1 in, 1 out]
                      }
                    }
                  }
                  frame True {
                  }
                }
              }
            }
          }
        }
      }
      event "Gasteiler löschen": Value Change {
        n158 = event-data() -> ()  [unwired: 1 in, 1 out]
        n159 = call "Texte in VIs uebersetzen.vi"("Sprachliste"=w218, "String zum Übersetzen"="Markierten Gasteiler wirklich löschen?" ("Nachricht")) -> ("String zum Übersetzen"=w225:string)  [unwired: 9 in, 4 out]
        n160 = call "Texte in VIs uebersetzen.vi"("Sprachliste"=w218, "String zum Übersetzen"="Ja" ("Text für T-Schaltfläche (\"OK\")")) -> ("String zum Übersetzen"=w224:string)  [unwired: 9 in, 4 out]
        n161 = call "Texte in VIs uebersetzen.vi"("Sprachliste"=w218, "String zum Übersetzen"="Nein" ("Text für F-Schaltfläche (\"Abbrechen\")")) -> ("String zum Übersetzen"=w223:string)  [unwired: 9 in, 4 out]
        n162 = Two Button Dialog(message=w225, 1:w223, 2:w224) -> (T button?=w219:bool)
        n163 = case shown="True" w219 {
          tunnel: w218 -> [_ w226]
          frame False {
          }
          frame True {
            w230 = ""
            n164 = local read "Gasteiler Tabelle"() -> (w235:i32)
            n165 = call "FGV SystemEinstellungenV2.vi"("Aktion"=Aktion_FGV_SystemEinstellungenV2."lesen") -> ("Gasteiler"=w228:T20)  [unwired: 5 in, 5 out]
            n166 = Unbundle By Name(w228) -> ("GasteilerDefinitionsListe"=w232:T19[])
            n167 = Get Date/Time In Seconds() -> (seconds since 1Jan1904=w229:timestamp)
            n168 = Index Array(array=w232, index=w235) -> (element=w227:T19)
            n169 = local write "Gasteiler Name"(w230) -> ()
            n170 = local write "Gasteiler Seriennummer"(w230) -> ()
            n171 = local write "Gasteiler Type"(w230) -> ()
            n172 = local write "Gasteiler Letzte Wartung"(w229) -> ()
            n173 = call "FGV SystemEinstellungenV2.vi"("Aktion"=Aktion_FGV_SystemEinstellungenV2."Gasteiler löschen", "Gasteiler definition"=w227) -> ("error out"=w233:errorcluster, "Gasteiler"=w231:T20)  [unwired: 4 in, 4 out]
            n174 = case shown="Fehler .." w233 {
              selector: w233 -> [_ w245]
              tunnel: w231 -> [w238 _]
              tunnel: w226 -> [_ w242]
              frame No Error {
                n175 = Unbundle By Name(w238) -> ("GasteilerDefinitionTextliste"=w237:string[][])
                n176 = call "FGV SystemEinstellungenV2.vi"("Aktion"=Aktion_FGV_SystemEinstellungenV2."speichern") -> ("error out"=w240:errorcluster)  [unwired: 5 in, 5 out]
                n177 = property on="Gasteiler Tabelle" class="MehrSpaltFeld (strikt)"(error in=w240, "ItemNames"=w237) -> (error out=w239:errorcluster)  [unwired: 1 in, 1 out]
                n178 = call <vilib>:"Clear Errors.vi"("error in (no error)"=w239) -> ()  [unwired: 5 in, 2 out]
              }
              frame Error {
                n179 = Unbundle By Name(w245) -> ("source"=w244:string)
                n180 = call "Texte in VIs uebersetzen.vi"("Sprachliste"=w242, "String zum Übersetzen"=w244) -> ("String zum Übersetzen"=w243:string)  [unwired: 9 in, 4 out]
                n181 = One Button Dialog(message=w243) -> ()  [unwired: 1 in, 1 out]
              }
            }
          }
        }
      }
      event "Neuer Gasteiler": Value Change {
        n182 = event-data() -> ()  [unwired: 1 in, 6 out]
        n183 = local read "Gasteiler Letzte Wartung"() -> (w247:timestamp)
        n184 = local read "Gasteiler Seriennummer"() -> (w248:string)
        n185 = local read "Gasteiler Type"() -> (w249:string)
        n186 = Empty String/Path?(string/path="Gasteiler Name") -> (empty?=w254:bool)
        n187 = Empty String/Path?(string/path=w249) -> (empty?=w255:bool)
        n188 = Select(t=w249, s=w254, f="Gasteiler Name") -> (s? t:f=w252:string)
        n189 = Select(t="Gasteiler Name", s=w255, f=w249) -> (s? t:f=w251:string)
        n190 = Empty String/Path?(string/path=w252) -> (empty?=w253:bool)
        n191 = case shown="False" w253 {
          tunnel: w252 -> [w264 _]
          tunnel: w251 -> [w263 _]
          tunnel: w248 -> [w262 _]
          tunnel: w247 -> [w261 _]
          tunnel: w246 -> [w257 _]
          frame False {
            n192 = Bundle("Gasteiler Name"=w264, "Gasteiler Type"=w263, "Gasteiler Seriennummer"=w262, "Gasteiler Letzte Wartung"=w261) -> (w260:T24)  [unwired: 1 in]
            n193 = call "FGV SystemEinstellungenV2.vi"("Aktion"=Aktion_FGV_SystemEinstellungenV2."Gasteiler schreiben", "Gasteiler definition"=w260) -> ("error out"=w256:errorcluster, "Gasteiler"=w258:T20, "Index Neuer Gasteiler"=w259:i32)  [unwired: 4 in, 3 out]
            n194 = case shown="Fehler .." w256 {
              selector: w256 -> [_ w278]
              tunnel: w258 -> [w267 _]
              tunnel: w259 -> [w266 _]
              tunnel: w257 -> [_ w275]
              frame No Error {
                n195 = stacked-sequence {
                  tunnel: w267 -> [w269 _]
                  tunnel: w266 -> [_ w274]
                  frame #0 {
                    n196 = Unbundle By Name(w269) -> ("GasteilerDefinitionTextliste"=w268:string[][])
                    n197 = call "FGV SystemEinstellungenV2.vi"("Aktion"=Aktion_FGV_SystemEinstellungenV2."speichern") -> ("error out"=w271:errorcluster)  [unwired: 5 in, 5 out]
                    n198 = property on="Gasteiler Tabelle" class="MehrSpaltFeld (strikt)"(error in=w271, "ItemNames"=w268) -> (error out=w270:errorcluster)  [unwired: 1 in, 1 out]
                    n199 = call <vilib>:"Clear Errors.vi"("error in (no error)"=w270) -> ()  [unwired: 5 in, 2 out]
                  }
                  frame #1 {
                    n200 = property on="Gasteiler Tabelle" class="MehrSpaltFeld (strikt)"("Val(Sgnl)"=w274) -> (error out=w273:errorcluster)  [unwired: 2 in, 1 out]
                    n201 = call <vilib>:"Clear Errors.vi"("error in (no error)"=w273) -> ()  [unwired: 5 in, 2 out]
                  }
                }
              }
              frame Error {
                n202 = Unbundle By Name(w278) -> ("source"=w277:string)
                n203 = call "Texte in VIs uebersetzen.vi"("Sprachliste"=w275, "String zum Übersetzen"=w277) -> ("String zum Übersetzen"=w276:string)  [unwired: 9 in, 4 out]
                n204 = One Button Dialog(message=w276) -> ()  [unwired: 1 in, 1 out]
              }
            }
          }
          frame True {
          }
        }
      }
      event "Analysatoren Liste": Value Change {
        n205 = event-data() -> ()  [unwired: 1 in, 1 out]
        n206 = call "FGV SystemEinstellungenV2.vi"("Aktion"=Aktion_FGV_SystemEinstellungenV2."lesen") -> ("Analysatoren"=w286:T23)  [unwired: 5 in, 5 out]
        n207 = Unbundle By Name(w286) -> ("AnalysatorDefinitionListe"=w283:T21[])
        n208 = Index Array(array=w283, index="Analysatoren Liste") -> (element=w284:T21)
        n209 = Unbundle By Name(w284) -> ("Analysator"=w280:string, "Name für Protokoll"=w282:string, "Seriennummer"=w281:string, "Type"=w279:string)
        n210 = local write "Analysator"(w280) -> ()
        n211 = local write "Name für Protokoll"(w282) -> ()
        n212 = local write "Seriennummer"(w281) -> ()
        n213 = local write "Type number (for Protocol)"(w279) -> ()
      }
      event "Analysator löschen": Value Change {
        n214 = event-data() -> ()  [unwired: 1 in, 1 out]
        n215 = call "Texte in VIs uebersetzen.vi"("Sprachliste"=w288, "String zum Übersetzen"="Markierten Analysator wirklich löschen?" ("Nachricht")) -> ("String zum Übersetzen"=w291:string)  [unwired: 9 in, 4 out]
        n216 = call "Texte in VIs uebersetzen.vi"("Sprachliste"=w288, "String zum Übersetzen"="Ja" ("Text für T-Schaltfläche (\"OK\")")) -> ("String zum Übersetzen"=w290:string)  [unwired: 9 in, 4 out]
        n217 = call "Texte in VIs uebersetzen.vi"("Sprachliste"=w288, "String zum Übersetzen"="Nein" ("Text für F-Schaltfläche (\"Abbrechen\")")) -> ("String zum Übersetzen"=w289:string)  [unwired: 9 in, 4 out]
        n218 = Two Button Dialog(message=w291, 1:w289, 2:w290) -> (T button?=w295:bool)
        n219 = case shown="True" w295 {
          frame False {
          }
          frame True {
            w297 = ""
            n220 = call "FGV SystemEinstellungenV2.vi"("Aktion"=Aktion_FGV_SystemEinstellungenV2."lesen") -> ("Analysatoren"=w299:T23)  [unwired: 5 in, 5 out]
            n221 = Unbundle By Name(w299) -> ("AnalysatorDefinitionListe"=w298:T21[])
            n222 = local read "Analysatoren Liste"() -> (w302:i32)
            n223 = Index Array(array=w298, index=w302) -> (element=w300:T21)
            n224 = local write "Type number (for Protocol)"(w297) -> ()
            n225 = local write "Seriennummer"(w297) -> ()
            n226 = local write "Name für Protokoll"(w297) -> ()
            n227 = call "FGV SystemEinstellungenV2.vi"("Aktion"=Aktion_FGV_SystemEinstellungenV2."Analysatoren löschen", "AnalysatorDefinition"=w300) -> ("error out"=w296:errorcluster)  [unwired: 4 in, 5 out]
            n228 = case shown="Fehler .." w296 {
              selector: w296 -> [_ w309]
              frame No Error {
                n229 = call "FGV SystemEinstellungenV2.vi"("Aktion"=Aktion_FGV_SystemEinstellungenV2."speichern") -> ("error out"=w307:errorcluster, "Analysatoren"=w304:T23)  [unwired: 5 in, 4 out]
                n230 = Unbundle By Name(w304) -> ("AnalysatorDefinitionTextListe"=w305:string[][])
                n231 = property on="Analysatoren Liste" class="MehrSpaltFeld (strikt)"(error in=w307, "ItemNames"=w305) -> (error out=w306:errorcluster)  [unwired: 1 in, 1 out]
                n232 = call <vilib>:"Clear Errors.vi"("error in (no error)"=w306) -> ()  [unwired: 5 in, 2 out]
              }
              frame Error {
                n233 = Unbundle By Name(w309) -> ("source"=w310:string)
                n234 = One Button Dialog(message=w310) -> ()  [unwired: 1 in, 1 out]
              }
            }
          }
        }
      }
      event "Seriennummer", "Name für Protokoll", "Type number (for Protocol)": Value Change {
        n235 = event-data() -> ()  [unwired: 1 in, 1 out]
        n236 = call "FGV SystemEinstellungenV2.vi"("Aktion"=Aktion_FGV_SystemEinstellungenV2."lesen") -> ("Analysatoren"=w314:T23)  [unwired: 5 in, 5 out]
        n237 = Unbundle By Name(w314) -> ("AnalysatorDefinitionListe"=w313:T21[])
        n238 = for {
          tunnel: w313 -> [w320] mode=indexing
          tunnel: "Analysator" -> [w318]
          tunnel: [w317] -> w312
          stop <- w317 stop-if-true
          n239 = Unbundle By Name(w320) -> ("Analysator"=w319:string)
          n240 = Equal?(x=w318, y=w319) -> (x = y?=w317:bool)
        }
        n241 = case shown="True" w312 {
          tunnel: w316 -> [_ w329]
          tunnel: "Analysator" -> [_ w321]
          frame False {
          }
          frame True {
            n242 = call "Texte in VIs uebersetzen.vi"("Sprachliste"=w329, "String zum Übersetzen"="Änderungen speichern?" ("Nachricht")) -> ("String zum Übersetzen"=w323:string)  [unwired: 9 in, 4 out]
            n243 = call "Texte in VIs uebersetzen.vi"("Sprachliste"=w329, "String zum Übersetzen"="Ja" ("Text für T-Schaltfläche (\"OK\")")) -> ("String zum Übersetzen"=w324:string)  [unwired: 9 in, 4 out]
            n244 = call "Texte in VIs uebersetzen.vi"("Sprachliste"=w329, "String zum Übersetzen"="Nein" ("Text für F-Schaltfläche (\"Abbrechen\")")) -> ("String zum Übersetzen"=w325:string)  [unwired: 9 in, 4 out]
            n245 = Two Button Dialog(message=w323, 1:w325, 2:w324) -> (T button?=w322:bool)
            n246 = case shown="True" w322 {
              tunnel: w321 -> [_ w330]
              frame False {
              }
              frame True {
                n247 = Empty String/Path?(string/path="Name für Protokoll") -> (empty?=w334:bool)
                n248 = Select(t=w330, s=w334, f="Name für Protokoll") -> (s? t:f=w332:T5)
                n249 = Empty String/Path?(string/path=w330) -> (empty?=w335:bool)
                n250 = case shown="False" w335 {
                  tunnel: "Seriennummer" -> [w342 _]
                  tunnel: w332 -> [w343 _]
                  tunnel: w330 -> [w341 _]
                  tunnel: "Type number (for Protocol)" -> [w340 _]
                  frame False {
                    n251 = Bundle By Name(cluster=T21 {"Analysator"="", "Name für Protokoll"="", "Type"="", "Seriennummer"=""} ("AnalysatorDefinition"), "Analysator"=w341, "Name für Protokoll"=w343, "Seriennummer"=w342, "Type"=w340) -> (w338:T21)
                    n252 = call "FGV SystemEinstellungenV2.vi"("Aktion"=Aktion_FGV_SystemEinstellungenV2."Analysator ändern", "AnalysatorDefinition"=w338) -> ("error out"=w337:errorcluster, "Analysatoren"=w345:T23, "Index Neuer analysator"=w344:i32)  [unwired: 4 in, 3 out]
                    n253 = case shown="Kein Fehler" w337 {
                      selector: w337 -> [_ w356]
                      tunnel: w345 -> [w348 _]
                      tunnel: w344 -> [w347 _]
                      frame No Error {
                        n254 = stacked-sequence {
                          tunnel: w348 -> [w350 _]
                          tunnel: w347 -> [_ w355]
                          frame #0 {
                            n255 = Unbundle By Name(w350) -> ("AnalysatorDefinitionTextListe"=w349:string[][])
                            n256 = call "FGV SystemEinstellungenV2.vi"("Aktion"=Aktion_FGV_SystemEinstellungenV2."speichern") -> ("error out"=w351:errorcluster)  [unwired: 5 in, 5 out]
                            n257 = property on="Analysatoren Liste" class="MehrSpaltFeld (strikt)"(error in=w351, "ItemNames"=w349) -> (error out=w353:errorcluster)  [unwired: 1 in, 1 out]
                            n258 = call <vilib>:"Clear Errors.vi"("error in (no error)"=w353) -> ()  [unwired: 5 in, 2 out]
                          }
                          frame #1 {
                            n259 = property on="Analysatoren Liste" class="MehrSpaltFeld (strikt)"("Val(Sgnl)"=w355) -> (error out=w354:errorcluster)  [unwired: 2 in, 1 out]
                            n260 = call <vilib>:"Clear Errors.vi"("error in (no error)"=w354) -> ()  [unwired: 5 in, 2 out]
                          }
                        }
                      }
                      frame Error {
                        n261 = Unbundle By Name(w356) -> ("source"=w357:string)
                        n262 = One Button Dialog(message=w357) -> ()  [unwired: 1 in, 1 out]
                      }
                    }
                  }
                  frame True {
                  }
                }
              }
            }
          }
        }
      }
      event "Neuer Analysator": Value Change {
        n263 = event-data() -> ()  [unwired: 1 in, 1 out]
        n264 = local read "Type number (for Protocol)"() -> (w359:string)
        n265 = local read "Name für Protokoll"() -> (w361:string)
        n266 = local read "Seriennummer"() -> (w362:string)
        n267 = local read "Analysator"() -> (w360:T5)
        n268 = Empty String/Path?(string/path=w361) -> (empty?=w364:bool)
        n269 = Empty String/Path?(string/path=w360) -> (empty?=w365:bool)
        n270 = Select(t=w360, s=w364, f=w361) -> (s? t:f=w363:T5)
        n271 = case shown="False" w365 {
          tunnel: w362 -> [w371 _]
          tunnel: w363 -> [w372 _]
          tunnel: w360 -> [w369 _]
          tunnel: w359 -> [w368 _]
          tunnel: w358 -> [w366 _]
          frame False {
            n272 = Bundle By Name(cluster=T21 {"Analysator"="", "Name für Protokoll"="", "Type"="", "Seriennummer"=""} ("AnalysatorDefinition"), "Analysator"=w369, "Name für Protokoll"=w372, "Seriennummer"=w371, "Type"=w368) -> (w370:T21)
            n273 = call "FGV SystemEinstellungenV2.vi"("Aktion"=Aktion_FGV_SystemEinstellungenV2."Analysatoren schreiben", "AnalysatorDefinition"=w370) -> ("error out"=w367:errorcluster, "Analysatoren"=w375:T23, "Index Neuer analysator"=w374:i32)  [unwired: 4 in, 3 out]
            n274 = case shown="Fehler .." w367 {
              selector: w367 -> [_ w389]
              tunnel: w375 -> [w378 _]
              tunnel: w374 -> [w377 _]
              tunnel: w366 -> [_ w388]
              frame No Error {
                n275 = stacked-sequence {
                  tunnel: w378 -> [w380 _]
                  tunnel: w377 -> [_ w385]
                  frame #0 {
                    n276 = Unbundle By Name(w380) -> ("AnalysatorDefinitionTextListe"=w379:string[][])
                    n277 = call "FGV SystemEinstellungenV2.vi"("Aktion"=Aktion_FGV_SystemEinstellungenV2."speichern") -> ("error out"=w381:errorcluster)  [unwired: 5 in, 5 out]
                    n278 = property on="Analysatoren Liste" class="MehrSpaltFeld (strikt)"(error in=w381, "ItemNames"=w379) -> (error out=w383:errorcluster)  [unwired: 1 in, 1 out]
                    n279 = call <vilib>:"Clear Errors.vi"("error in (no error)"=w383) -> ()  [unwired: 5 in, 2 out]
                  }
                  frame #1 {
                    n280 = property on="Analysatoren Liste" class="MehrSpaltFeld (strikt)"("Val(Sgnl)"=w385) -> (error out=w384:errorcluster)  [unwired: 2 in, 1 out]
                    n281 = call <vilib>:"Clear Errors.vi"("error in (no error)"=w384) -> ()  [unwired: 5 in, 2 out]
                  }
                }
              }
              frame Error {
                n282 = Unbundle By Name(w389) -> ("source"=w387:string)
                n283 = call "Texte in VIs uebersetzen.vi"("Sprachliste"=w388, "String zum Übersetzen"=w387) -> ("String zum Übersetzen"=w386:string)  [unwired: 9 in, 4 out]
                n284 = One Button Dialog(message=w386) -> ()  [unwired: 1 in, 1 out]
              }
            }
          }
          frame True {
          }
        }
      }
      event "Update Gas Selects": Value Change {
        n285 = event-data() -> ()  [unwired: 1 in, 6 out]
        n286 = control-ref of="Gasauswahl"() -> (w390:refnum<vi>)
        n287 = control-ref of="Gasauswahl"() -> (w391:refnum<vi>)
        n288 = control-ref of="Gasauswahl"() -> (w392:refnum<vi>)
        n289 = control-ref of="Gasauswahl"() -> (w393:refnum<vi>)
        n290 = control-ref of="Gasauswahl"() -> (w394:refnum<vi>)
        n291 = Build Array(w390, w391, w392, w393, w394) -> (w395:refnum<vi>[])
        n292 = for {
          tunnel: w395 -> [w396] mode=indexing
          n293 = call "Gasauswahl befuellen.vi"("Kombinationsfeld (Eingang)"=w396) -> ()  [unwired: 11 in]
        }
      }
      event "Gasflaschenliste löschen": Value Change {
        n294 = event-data() -> ()  [unwired: 1 in, 1 out]
        n295 = call "Texte in VIs uebersetzen.vi"("Sprachliste"=w397, "String zum Übersetzen"="Gesamte Gasflaschenliste wirklich löschen?" ("Nachricht")) -> ("String zum Übersetzen"=w399:string)  [unwired: 9 in, 4 out]
        n296 = call "Texte in VIs uebersetzen.vi"("Sprachliste"=w397, "String zum Übersetzen"="Ja" ("Text für T-Schaltfläche (\"OK\")")) -> ("String zum Übersetzen"=w400:string)  [unwired: 9 in, 4 out]
        n297 = call "Texte in VIs uebersetzen.vi"("Sprachliste"=w397, "String zum Übersetzen"="Nein" ("Text für F-Schaltfläche (\"Abbrechen\")")) -> ("String zum Übersetzen"=w401:string)  [unwired: 9 in, 4 out]
        n298 = Two Button Dialog(message=w399, 1:w401, 2:w400) -> (T button?=w398:bool)
        n299 = case shown="True" w398 {
          tunnel: w397 -> [_ w405]
          frame False {
          }
          frame True {
            n300 = Bundle By Name(cluster=T7 {"Gasauswahl"="NH3", "Konzentration IST"=2000.0, "Einheit"="ppm", "Genauigkeit"=2.0} ("Komponente 1"), "Gasauswahl"="", "Konzentration IST"=0.0) -> (w412:T7)
            n301 = property on="Gasflaschen Liste" class="MehrSpaltFeld (strikt)"() -> ("ItemNames"=w406:string[][])  [unwired: 2 in, 2 out]
            n302 = local write "Komponente 1"(w412) -> ()
            n303 = local write "Komponente 2"(w412) -> ()
            n304 = local write "Komponente 3"(w412) -> ()
            n305 = local write "Komponente 4"(w412) -> ()
            n306 = local write "Komponente 5"(w412) -> ()
            n307 = for {
              tunnel: [w419] -> w407
              tunnel: w406 -> [w417] mode=indexing
              n308 = call "FGV Gasbottledefinition.vi"("Aktion"=Aktion_FGV_Gasbottledefinition."löschen", "Gasflasche Text Array"=w417) -> ("error out"=w419:errorcluster)  [unwired: 7 in, 2 out]
            }
            n309 = Get Date/Time In Seconds() -> (seconds since 1Jan1904=w410:timestamp)
            n310 = case shown="Fehler .." w407 {
              selector: w407 -> [_ w428]
              tunnel: w405 -> [_ w425]
              frame No Error {
                n311 = call "FGV Gasbottledefinition.vi"("Aktion"=Aktion_FGV_Gasbottledefinition."speichern") -> ("error out"=w423:errorcluster, "Gasflaschen Text Liste gesamt"=w422:T6[][])  [unwired: 8 in, 1 out]
                n312 = property on="Gasflaschen Liste" class="MehrSpaltFeld (strikt)"(error in=w423, "ItemNames"=w422, "Value"=-1 ("Gasflaschen Liste")) -> (error out=w421:errorcluster)  [unwired: 1 in, 1 out]
                n313 = call <vilib>:"Clear Errors.vi"("error in (no error)"=w421) -> ()  [unwired: 5 in, 2 out]
              }
              frame Error {
                n314 = Unbundle By Name(w428) -> ("source"=w427:string)
                n315 = call "Texte in VIs uebersetzen.vi"("Sprachliste"=w425, "String zum Übersetzen"=w427) -> ("String zum Übersetzen"=w426:string)  [unwired: 9 in, 4 out]
                n316 = One Button Dialog(message=w426) -> ()  [unwired: 1 in, 1 out]
              }
            }
            n317 = local write "Gasflaschenliste löschen"(FALSE ("Gasflaschen Maske leeren")) -> ()
            n318 = Bundle By Name(cluster=T8 {"Gasname für die Auswahl"="", "Chargennummer"="", "Ablaufdatum"=timestamp(3724444800 s since 1904-01-01)} ("Gasflasche"), "Ablaufdatum"=w410) -> (w411:T8)
            n319 = local write "Gasflasche"(w411) -> ()
            n320 = local write "Trägergas"(T6 "N2" ("Trägergas")) -> ()
          }
        }
      }
      event "Gas löschen": Value Change {
        n321 = event-data() -> ()  [unwired: 1 in, 1 out]
        n322 = call "Texte in VIs uebersetzen.vi"("Sprachliste"=w429, "String zum Übersetzen"="Markiertes Gas wirklich löschen?" ("Nachricht")) -> ("String zum Übersetzen"=w436:string)  [unwired: 9 in, 4 out]
        n323 = call "Texte in VIs uebersetzen.vi"("Sprachliste"=w429, "String zum Übersetzen"="Ja" ("Text für T-Schaltfläche (\"OK\")")) -> ("String zum Übersetzen"=w435:string)  [unwired: 9 in, 4 out]
        n324 = call "Texte in VIs uebersetzen.vi"("Sprachliste"=w429, "String zum Übersetzen"="Nein" ("Text für F-Schaltfläche (\"Abbrechen\")")) -> ("String zum Übersetzen"=w434:string)  [unwired: 9 in, 4 out]
        n325 = Two Button Dialog(message=w436, 1:w434, 2:w435) -> (T button?=w430:bool)
        n326 = case shown="True" w430 {
          tunnel: w429 -> [_ w437]
          frame False {
          }
          frame True {
            n327 = property on="Gasauswahl" class="Listenfeld (strikt)"() -> (error out=w440:errorcluster, "Value"=w442:i32)  [unwired: 2 in, 1 out]
            n328 = property on="Gasauswahl" class="Listenfeld (strikt)"(error in=w440) -> ("Item Names"=w443:string[])  [unwired: 1 in, 2 out]
            n329 = Index Array(array=w443, index=w442) -> (element=w441:string)
            n330 = call "FGV Gasdefinition.vi"("Aktion"=T14."löschen", "Gas"=w441) -> ("error out"=w438:errorcluster, "Gase"=w439:string[])  [unwired: 8 in]
            n331 = case shown="Fehler .." w438 {
              selector: w438 -> [_ w455]
              tunnel: w439 -> [w451 _]
              tunnel: w437 -> [_ w452]
              frame No Error {
                n332 = call "FGV Gasdefinition.vi"("Aktion"=T14."speichern") -> ("error out"=w448:errorcluster)  [unwired: 9 in, 1 out]
                n333 = property on="Gasauswahl" class="Listenfeld (strikt)"(error in=w448, "Item Names"=w451, "Value"=-1 ("Gasauswahl")) -> (error out=w447:errorcluster)  [unwired: 1 in, 1 out]
                n334 = property on="Update Gas Selects" class="Bool. (strikt)"(error in=w447, "Val(Sgnl)"=TRUE ("Wert (signalisierend)")) -> (error out=w446:errorcluster)  [unwired: 1 in, 1 out]
                n335 = call <vilib>:"Clear Errors.vi"("error in (no error)"=w446) -> ()  [unwired: 5 in, 2 out]
              }
              frame Error {
                n336 = Unbundle By Name(w455) -> ("source"=w454:string)
                n337 = call "Texte in VIs uebersetzen.vi"("Sprachliste"=w452, "String zum Übersetzen"=w454) -> ("String zum Übersetzen"=w453:string)  [unwired: 9 in, 4 out]
                n338 = One Button Dialog(message=w453) -> ()  [unwired: 1 in, 1 out]
              }
            }
          }
        }
      }
      event "Gas einfügen": Value Change {
        n339 = event-data() -> ()  [unwired: 1 in, 1 out]
        n340 = call "FGV Gasdefinition.vi"("Aktion"=T14."schreiben", "Gas"="Gas Eingabe") -> ("error out"=w457:errorcluster, "Gase"=w458:string[])  [unwired: 8 in]
        n341 = case shown="Fehler .." w457 {
          selector: w457 -> [_ w471]
          tunnel: w458 -> [w467 _]
          tunnel: w456 -> [_ w468]
          frame No Error {
            n342 = call "FGV Gasdefinition.vi"("Aktion"=T14."speichern") -> ("error out"=w464:errorcluster)  [unwired: 9 in, 1 out]
            n343 = property on="Gasauswahl" class="Listenfeld (strikt)"(error in=w464, "Item Names"=w467, "Value"=-1 ("Gasauswahl")) -> (error out=w463:errorcluster)  [unwired: 1 in, 1 out]
            n344 = property on="Update Gas Selects" class="Bool. (strikt)"(error in=w463, "Val(Sgnl)"=TRUE ("Wert (signalisierend)")) -> (error out=w462:errorcluster)  [unwired: 1 in, 1 out]
            n345 = call <vilib>:"Clear Errors.vi"("error in (no error)"=w462) -> ()  [unwired: 5 in, 2 out]
          }
          frame Error {
            n346 = Unbundle By Name(w471) -> ("source"=w470:string)
            n347 = call "Texte in VIs uebersetzen.vi"("Sprachliste"=w468, "String zum Übersetzen"=w470) -> ("String zum Übersetzen"=w469:string)  [unwired: 9 in, 4 out]
            n348 = One Button Dialog(message=w469) -> ()  [unwired: 1 in, 1 out]
          }
        }
      }
      event "Gasauswahl": Double Click {
        n349 = event-data() -> ()  [unwired: 1 in, 9 out]
        n350 = property on="Gasauswahl" class="Listenfeld (strikt)"() -> (error out=w473:errorcluster, "Value"=w475:i32)  [unwired: 2 in, 1 out]
        n351 = property on="Gasauswahl" class="Listenfeld (strikt)"(error in=w473) -> (error out=w472:errorcluster, "Item Names"=w476:string[])  [unwired: 1 in, 1 out]
        n352 = Index Array(array=w476, index=w475) -> (element=w474:string)
        n353 = call <vilib>:"Clear Errors.vi"("error in (no error)"=w472) -> ()  [unwired: 5 in, 2 out]
        n354 = local write "Gas Eingabe"(w474) -> ()
      }
      event "Gasflaschen Liste": Value Change {
        n355 = event-data() -> ()  [unwired: 1 in, 1 out]
        n356 = property on="Gasflaschen Liste" class="MehrSpaltFeld (strikt)"() -> ("ItemNames"=w488:string[][], "Value"=w487:i32)  [unwired: 2 in, 2 out]
        n357 = Index Array(array=w488, index (row)=w487) -> (element=w486:string[])  [unwired: 1 in]
        n358 = call "Gasflasche Text in Cluster.vi"("Gasflasche Text Array"=w486) -> ("Gasflasche"=w485:T25)  [unwired: 10 in]
        n359 = Unbundle By Name(w485) -> ("Gasflasche"=w484:T8, "Trägergas"=w483:T6, "Komponenten"=w482:T7[])
        n360 = Index Array(array=w482) -> (element #1=w481:T7, element #2=w480:T7, element #3=w479:T7, element #4=w478:T7, element #5=w477:T7)  [unwired: 5 in]
        n361 = local write "Gasflasche"(w484) -> ()
        n362 = local write "Trägergas"(w483) -> ()
        n363 = local write "Komponente 1"(w481) -> ()
        n364 = local write "Komponente 2"(w480) -> ()
        n365 = local write "Komponente 3"(w479) -> ()
        n366 = local write "Komponente 4"(w478) -> ()
        n367 = local write "Komponente 5"(w477) -> ()
      }
      event "GF export": Value Change {
        n368 = event-data() -> ()  [unwired: 1 in, 6 out]
        n369 = call "FGV Gasbottledefinition.vi"("Aktion"=Aktion_FGV_Gasbottledefinition."speichern") -> ("error out"=w491:errorcluster)  [unwired: 8 in, 2 out]
        n370 = call "FGV Gasbottledefinition.vi"("Aktion"=Aktion_FGV_Gasbottledefinition."exportieren", "error in (no error)"=w491) -> ("error out"=w490:errorcluster)  [unwired: 7 in, 2 out]
        n371 = case shown="Kein Fehler" w490 {
          tunnel: w489 -> [w494 w498]
          frame No Error {
            n372 = call "Texte in VIs uebersetzen.vi"("Sprachliste"=w494, "String zum Übersetzen"="Gasflaschenliste exportiert!" ("Nachricht")) -> ("String zum Übersetzen"=w497:string)  [unwired: 9 in, 4 out]
            n373 = One Button Dialog(message=w497, button name ("OK")="OK" ("Schaltflächentext (\"OK\")")) -> ()  [unwired: 1 out]
          }
          frame Error {
            n374 = call "Texte in VIs uebersetzen.vi"("Sprachliste"=w498, "String zum Übersetzen"="Fehler beim Exportieren!" ("Nachricht")) -> ("String zum Übersetzen"=w501:string)  [unwired: 9 in, 4 out]
            n375 = One Button Dialog(message=w501, button name ("OK")="OK" ("Schaltflächentext (\"OK\")")) -> ()  [unwired: 1 out]
          }
        }
      }
      event "GF import": Value Change {
        n376 = event-data() -> ()  [unwired: 1 in, 1 out]
        n377 = call "FGV Gasbottledefinition.vi"("Aktion"=Aktion_FGV_Gasbottledefinition."importieren") -> ("error out"=w503:errorcluster)  [unwired: 8 in, 2 out]
        n378 = case shown="Kein Fehler" w503 {
          tunnel: w502 -> [w508 w521]
          frame No Error {
            n379 = call "FGV Gasbottledefinition.vi"("Aktion"=Aktion_FGV_Gasbottledefinition."lesen") -> ("error out"=w512:errorcluster, "Gasflaschen Text Liste gesamt"=w519:T6[][])  [unwired: 8 in, 1 out]
            n380 = property on="Gasflaschen Liste" class="MehrSpaltFeld (strikt)"(error in=w512, "ItemNames"=w519, "Value"=-1 ("Gasflaschen Liste")) -> (error out=w515:errorcluster)  [unwired: 1 in, 1 out]
            n381 = call "FGV Gasdefinition.vi"("Aktion"=T14."lesen", "error in (no error)"=w512) -> ("Gase"=w516:string[])  [unwired: 8 in, 1 out]
            n382 = property on="Gasauswahl" class="Listenfeld (strikt)"(error in=w515, "Item Names"=w516) -> (error out=w514:errorcluster)  [unwired: 1 in, 1 out]
            n383 = call "Texte in VIs uebersetzen.vi"("Sprachliste"=w508, "String zum Übersetzen"="Gasflaschenliste importiert!" ("Nachricht")) -> ("String zum Übersetzen"=w511:string)  [unwired: 9 in, 4 out]
            n384 = property on="Update Gas Selects" class="Bool. (strikt)"(error in=w514, "Val(Sgnl)"=TRUE ("Wert (signalisierend)")) -> (error out=w507:errorcluster)  [unwired: 1 in, 1 out]
            n385 = One Button Dialog(message=w511, button name ("OK")="OK" ("Schaltflächentext (\"OK\")")) -> ()  [unwired: 1 out]
            n386 = call <vilib>:"Clear Errors.vi"("error in (no error)"=w507) -> ("error out"=w505:errorcluster)  [unwired: 5 in, 1 out]
            n387 = call "FGV Gasbottledefinition.vi"("Aktion"=Aktion_FGV_Gasbottledefinition."speichern", "error in (no error)"=w505) -> ()  [unwired: 7 in, 3 out]
          }
          frame Error {
            n388 = call "Texte in VIs uebersetzen.vi"("Sprachliste"=w521, "String zum Übersetzen"="Fehler beim Importieren!" ("Nachricht")) -> ("String zum Übersetzen"=w524:string)  [unwired: 9 in, 4 out]
            n389 = One Button Dialog(message=w524, button name ("OK")="OK" ("Schaltflächentext (\"OK\")")) -> ()  [unwired: 1 out]
          }
        }
      }
      event "Gasflasche einfügen": Value Change {
        n390 = event-data() -> ()  [unwired: 1 in, 1 out]
        n391 = Build Array("Komponente 1", "Komponente 2", "Komponente 3", "Komponente 4", "Komponente 5") -> (w531:T7[])
        n392 = Bundle("Gasflasche"="Gasflasche", "Trägergas"="Trägergas", w531) -> (w530:cluster{"Gasflasche":T8, "Trägergas":T6, T7[]})  [unwired: 1 in]
        n393 = call "Gasflasche Cluster in Text.vi"("Gasflasche"=w530) -> ("Gasflasche Text Array"=w528:T6[])  [unwired: 10 in]
        n394 = call "FGV Gasbottledefinition.vi"("Aktion"=Aktion_FGV_Gasbottledefinition."schreiben", "Gasflasche Text Array"=w528) -> ("error out"=w526:errorcluster, "Gasflaschen Text Liste gesamt"=w527:T6[][])  [unwired: 7 in, 1 out]
        n395 = case shown="Fehler .." w526 {
          selector: w526 -> [_ w546]
          tunnel: w527 -> [w541 _]
          tunnel: w525 -> [_ w543]
          frame No Error {
            n396 = call "FGV Gasbottledefinition.vi"("Aktion"=Aktion_FGV_Gasbottledefinition."speichern") -> ("error out"=w539:errorcluster)  [unwired: 8 in, 2 out]
            n397 = property on="Gasflaschen Liste" class="MehrSpaltFeld (strikt)"(error in=w539, "ItemNames"=w541) -> (error out=w540:errorcluster)  [unwired: 1 in, 1 out]
            n398 = call <vilib>:"Clear Errors.vi"("error in (no error)"=w540) -> ()  [unwired: 5 in, 2 out]
          }
          frame Error {
            n399 = Unbundle By Name(w546) -> ("source"=w545:string)
            n400 = call "Texte in VIs uebersetzen.vi"("Sprachliste"=w543, "String zum Übersetzen"=w545) -> ("String zum Übersetzen"=w544:string)  [unwired: 9 in, 4 out]
            n401 = One Button Dialog(message=w544) -> ()  [unwired: 1 in, 1 out]
          }
        }
      }
      event "Gasflasche ändern": Value Change {
        n402 = event-data() -> ()  [unwired: 1 in, 1 out]
        n403 = call "Texte in VIs uebersetzen.vi"("Sprachliste"=w547, "String zum Übersetzen"="Änderungen speichern?" ("Nachricht")) -> ("String zum Übersetzen"=w554:string)  [unwired: 9 in, 4 out]
        n404 = call "Texte in VIs uebersetzen.vi"("Sprachliste"=w547, "String zum Übersetzen"="Ja" ("Text für T-Schaltfläche (\"OK\")")) -> ("String zum Übersetzen"=w553:string)  [unwired: 9 in, 4 out]
        n405 = call "Texte in VIs uebersetzen.vi"("Sprachliste"=w547, "String zum Übersetzen"="Nein" ("Text für F-Schaltfläche (\"Abbrechen\")")) -> ("String zum Übersetzen"=w552:string)  [unwired: 9 in, 4 out]
        n406 = Two Button Dialog(message=w554, 1:w552, 2:w553) -> (T button?=w548:bool)
        n407 = case shown="True" w548 {
          tunnel: w547 -> [_ w555]
          frame False {
          }
          frame True {
            n408 = local read "Gasflasche"() -> (w568:T8)
            n409 = local read "Trägergas"() -> (w567:T6)
            n410 = local read "Komponente 1"() -> (w566:T7)
            n411 = local read "Komponente 2"() -> (w565:T7)
            n412 = local read "Komponente 3"() -> (w564:T7)
            n413 = local read "Komponente 4"() -> (w563:T7)
            n414 = local read "Komponente 5"() -> (w562:T7)
            n415 = property on="Gasflaschen Liste" class="MehrSpaltFeld (strikt)"() -> ("Value"=w559:i32, "ItemNames"=w558:string[][])  [unwired: 2 in, 2 out]
            n416 = Build Array(w566, w565, w564, w563, w562) -> (w561:T7[])
            n417 = Index Array(array=w558, index (row)=w559) -> (element=w560:string[])  [unwired: 1 in]
            n418 = Bundle("Gasflasche"=w568, "Trägergas"=w567, w561) -> (w570:cluster{"Gasflasche":T8, "Trägergas":T6, T7[]})  [unwired: 1 in]
            n419 = call "FGV Gasbottledefinition.vi"("Aktion"=T14."löschen", "Gasflasche Text Array"=w560) -> ("error out"=w556:errorcluster)  [unwired: 7 in, 2 out]
            n420 = call "Gasflasche Cluster in Text.vi"("Gasflasche"=w570) -> ("Gasflasche Text Array"=w569:T6[])  [unwired: 10 in]
            n421 = case shown="Fehler .." w556 {
              selector: w556 -> [_ w587]
              tunnel: w569 -> [w575 _]
              tunnel: w555 -> [w571 w584]
              frame No Error {
                n422 = call "FGV Gasbottledefinition.vi"("Aktion"=Aktion_FGV_Gasbottledefinition."schreiben", "Gasflasche Text Array"=w575) -> ("error out"=w573:errorcluster, "Gasflaschen Text Liste gesamt"=w574:T6[][])  [unwired: 7 in, 1 out]
                n423 = case shown="Fehler .." w573 {
                  selector: w573 -> [_ w583]
                  tunnel: w574 -> [w578 _]
                  tunnel: w571 -> [_ w580]
                  frame No Error {
                    n424 = call "FGV Gasbottledefinition.vi"("Aktion"=Aktion_FGV_Gasbottledefinition."speichern") -> ("error out"=w577:errorcluster)  [unwired: 8 in, 2 out]
                    n425 = property on="Gasflaschen Liste" class="MehrSpaltFeld (strikt)"(error in=w577, "ItemNames"=w578) -> (error out=w576:errorcluster)  [unwired: 1 in, 1 out]
                    n426 = call <vilib>:"Clear Errors.vi"("error in (no error)"=w576) -> ()  [unwired: 5 in, 2 out]
                  }
                  frame Error {
                    n427 = Unbundle By Name(w583) -> ("source"=w582:string)
                    n428 = call "Texte in VIs uebersetzen.vi"("Sprachliste"=w580, "String zum Übersetzen"=w582) -> ("String zum Übersetzen"=w581:string)  [unwired: 9 in, 4 out]
                    n429 = One Button Dialog(message=w581) -> ()  [unwired: 1 in, 1 out]
                  }
                }
              }
              frame Error {
                n430 = Unbundle By Name(w587) -> ("source"=w586:string)
                n431 = call "Texte in VIs uebersetzen.vi"("Sprachliste"=w584, "String zum Übersetzen"=w586) -> ("String zum Übersetzen"=w585:string)  [unwired: 9 in, 4 out]
                n432 = One Button Dialog(message=w585) -> ()  [unwired: 1 in, 1 out]
              }
            }
          }
        }
      }
      event "Gasflasche löschen": Value Change {
        n433 = event-data() -> ()  [unwired: 1 in, 1 out]
        n434 = call "Texte in VIs uebersetzen.vi"("Sprachliste"=w588, "String zum Übersetzen"="Markierte Gasflasche wirklich löschen?" ("Nachricht")) -> ("String zum Übersetzen"=w595:string)  [unwired: 9 in, 4 out]
        n435 = call "Texte in VIs uebersetzen.vi"("Sprachliste"=w588, "String zum Übersetzen"="Ja" ("Text für T-Schaltfläche (\"OK\")")) -> ("String zum Übersetzen"=w594:string)  [unwired: 9 in, 4 out]
        n436 = call "Texte in VIs uebersetzen.vi"("Sprachliste"=w588, "String zum Übersetzen"="Nein" ("Text für F-Schaltfläche (\"Abbrechen\")")) -> ("String zum Übersetzen"=w593:string)  [unwired: 9 in, 4 out]
        n437 = Two Button Dialog(message=w595, 1:w593, 2:w594) -> (T button?=w589:bool)
        n438 = case shown="True" w589 {
          tunnel: w588 -> [_ w596]
          frame False {
          }
          frame True {
            n439 = property on="Gasflaschen Liste" class="MehrSpaltFeld (strikt)"() -> ("Value"=w601:i32, "ItemNames"=w600:string[][])  [unwired: 2 in, 2 out]
            n440 = Index Array(array=w600, index (row)=w601) -> (element=w598:string[])  [unwired: 1 in]
            n441 = call "FGV Gasbottledefinition.vi"("Aktion"=Aktion_FGV_Gasbottledefinition."löschen", "Gasflasche Text Array"=w598) -> ("error out"=w597:errorcluster)  [unwired: 7 in, 2 out]
            n442 = case shown="Fehler .." w597 {
              selector: w597 -> [_ w610]
              tunnel: w596 -> [_ w607]
              frame No Error {
                n443 = call "FGV Gasbottledefinition.vi"("Aktion"=Aktion_FGV_Gasbottledefinition."speichern") -> ("error out"=w605:errorcluster, "Gasflaschen Text Liste gesamt"=w604:T6[][])  [unwired: 8 in, 1 out]
                n444 = property on="Gasflaschen Liste" class="MehrSpaltFeld (strikt)"(error in=w605, "ItemNames"=w604, "Value"=-1 ("Gasflaschen Liste")) -> (error out=w603:errorcluster)  [unwired: 1 in, 1 out]
                n445 = call <vilib>:"Clear Errors.vi"("error in (no error)"=w603) -> ()  [unwired: 5 in, 2 out]
              }
              frame Error {
                n446 = Unbundle By Name(w610) -> ("source"=w609:string)
                n447 = call "Texte in VIs uebersetzen.vi"("Sprachliste"=w607, "String zum Übersetzen"=w609) -> ("String zum Übersetzen"=w608:string)  [unwired: 9 in, 4 out]
                n448 = One Button Dialog(message=w608) -> ()  [unwired: 1 in, 1 out]
              }
            }
          }
        }
      }
      event "Gasteiler Importieren": Value Change {
        n449 = event-data() -> ()  [unwired: 1 in, 1 out]
        n450 = call "FGV SystemEinstellungenV2.vi"("Aktion"=Aktion_FGV_SystemEinstellungenV2."Gasteiler importieren") -> ("Gasteiler"=w613:T20)  [unwired: 5 in, 5 out]
        n451 = Unbundle By Name(w613) -> ("GasteilerDefinitionTextliste"=w612:string[][])
        n452 = property on="Gasteiler Tabelle" class="MehrSpaltFeld (strikt)"("ItemNames"=w612) -> (error out=w611:errorcluster)  [unwired: 2 in, 1 out]
        n453 = call <vilib>:"Clear Errors.vi"("error in (no error)"=w611) -> ()  [unwired: 5 in, 2 out]
      }
      event "Gasteiler Export": Value Change {
        n454 = event-data() -> ()  [unwired: 1 in, 1 out]
        n455 = call "FGV SystemEinstellungenV2.vi"("Aktion"=Aktion_FGV_SystemEinstellungenV2."Gasteiler exportieren") -> ("error out"=w616:errorcluster)  [unwired: 5 in, 5 out]
        n456 = case shown="Fehler .." w616 {
          tunnel: w615 -> [w618 w622]
          frame No Error {
            n457 = call "Texte in VIs uebersetzen.vi"("Sprachliste"=w618, "String zum Übersetzen"="Gasteilerliste exportiert!" ("Nachricht")) -> ("String zum Übersetzen"=w621:string)  [unwired: 9 in, 4 out]
            n458 = One Button Dialog(message=w621, button name ("OK")="OK" ("Schaltflächentext (\"OK\")")) -> ()  [unwired: 1 out]
          }
          frame Error {
            n459 = call "Texte in VIs uebersetzen.vi"("Sprachliste"=w622, "String zum Übersetzen"="Fehler beim Exportieren!" ("Nachricht")) -> ("String zum Übersetzen"=w625:string)  [unwired: 9 in, 4 out]
            n460 = One Button Dialog(message=w625, button name ("OK")="OK" ("Schaltflächentext (\"OK\")")) -> ()  [unwired: 1 out]
          }
        }
      }
    }
  }
